vi "UFF_58.vi"(11 "array":string[](array[string])=["    58", "Transfer Function H1", "Vib & Ref1  H1 Velocity / Force", "25-Jul-01 16-14-15  ", "rubblkbrftn.svd", "NONE", "    4         3    1         0       NONE       513   2       NONE       501   2", "         5      3200         1  1.25000e+00  1.25000e+00  0.00000e+00", "        18    0    0    0            Frequency                   Hz", "        11    0    0    0             Velocity                  m/s", "        13    0    0    0                Force                    N", "         0    0    0    0                 NONE                 NONE", " -2.44772e-02 -2.29083e-02 -4.29675e-02 -3.38422e-02 -1.42753e-02 -1.87575e-02", " -4.10837e-02 -9.69093e-02 -2.05625e-01 -1.49768e-01 -3.44395e-01  1.65721e-01", " -1.09695e-01  3.16244e-01  2.64647e-01 -3.79660e-01 -3.12266e-02  6.21503e-02", " -3.37903e-02  5.86053e-02 -1.27031e-02  7.12610e-02  8.31891e-03  5.38217e-02", "  2.07081e-02  4.42556e-02  1.68963e-02  2.46244e-02  2.45377e-04 -1.47570e-02", " -5.97549e-02  3.47108e-02 -1.52918e-02  4.27029e-02 -1.50761e-02  4.24537e-02", " -5.81629e-03  3.90005e-02 -9.52282e-03  2.12302e-02 -1.48471e-02  3.79965e-02", " -6.36889e-03  4.28727e-02  1.19483e-03  3.87167e-02 -5.26405e-03  2.65269e-02", " -6.60730e-03  3.47906e-02  7.59866e-04  3.38277e-02 -1.54237e-03  3.24441e-02", "  1.03543e-03  3.03496e-02  3.38132e-03  3.12400e-02  6.82404e-03  2.80844e-02", "  6.40410e-03  2.41087e-02  4.76068e-03  2.30825e-02  4.81669e-03  2.17997e-02", "  4.57283e-03  2.07062e-02  4.58951e-03  1.95397e-02  4.21995e-03  1.79763e-02", "  3.77206e-03  1.86075e-02  3.65505e-03  1.45262e-02  8.31854e-03  1.77252e-02", "  4.44066e-04  1.54022e-02  2.11637e-03  1.37485e-02  1.98206e-03  1.44290e-02", "  8.26905e-04  1.30683e-02  8.12047e-04  1.29353e-02  9.44722e-04  1.27583e-02", "  7.80146e-04  1.20994e-02  6.20840e-04  1.14556e-02  1.53683e-04  1.13300e-02", " -1.26091e-04  1.08185e-02 -4.79234e-05  1.05322e-02 -2.48779e-04  1.01732e-02", " -2.57901e-04  9.65408e-03 -2.34030e-04  9.21830e-03 -6.76051e-04  8.78385e-03", " -4.73517e-04  8.30843e-03 -6.25769e-04  7.97665e-03 -8.67610e-04  7.67506e-03", " -8.06777e-04  7.30798e-03 -8.69391e-04  6.83099e-03 -1.08317e-03  6.43512e-03", " -1.04846e-03  6.14125e-03 -1.11451e-03  5.65235e-03 -1.40155e-03  5.38275e-03", " -1.08489e-03  5.29333e-03 -1.25805e-03  4.60217e-03 -1.34644e-03  4.25631e-03", " -1.42998e-03  3.83266e-03 -1.58892e-03  3.48706e-03 -1.49756e-03  3.32678e-03", " -1.65587e-03  2.96426e-03 -1.45823e-03  2.70408e-03 -1.36304e-03  2.35338e-03", " -1.40112e-03  2.03333e-03 -1.35197e-03  1.67269e-03 -1.33700e-03  1.33033e-03", " -1.38712e-03  1.02474e-03 -1.35330e-03  7.04625e-04 -1.34168e-03  3.02493e-04", " -1.31492e-03  4.42537e-05 -1.24354e-03 -2.61606e-04 -1.31045e-03 -5.85098e-04", " -1.23041e-03 -8.40868e-04 -1.19052e-03 -1.14186e-03 -1.15886e-03 -1.45960e-03", " -1.13493e-03 -1.81665e-03 -1.19200e-03 -2.09698e-03 -1.17228e-03 -2.32472e-03", " -1.13574e-03 -2.58351e-03 -1.05089e-03 -2.89408e-03 -1.02939e-03 -3.20176e-03", " -1.01978e-03 -3.53409e-03 -1.05770e-03 -3.85076e-03 -1.01618e-03 -4.15908e-03", " -1.05827e-03 -4.51371e-03 -1.05969e-03 -4.91698e-03 -1.11136e-03 -5.40058e-03", " -1.33444e-03 -6.24271e-03 -2.02819e-03 -7.93219e-03 -1.20950e-02 -1.05859e-02", " -1.23938e-03 -7.21660e-04 -5.88633e-04 -3.52608e-03 -6.26043e-04 -4.70434e-03", " -6.49080e-04 -5.59269e-03 -7.90585e-04 -6.39017e-03 -1.05691e-03 -7.20279e-03", " -1.49888e-03 -8.30801e-03 -2.48368e-03 -1.00025e-02 -5.73948e-03 -1.28778e-02", " -2.03627e-02 -1.04256e-02 -6.41621e-03  7.27220e-03 -1.12501e-03  1.48627e-03", " -3.76965e-04 -1.26116e-03 -1.63673e-04 -2.42729e-03 -1.05605e-04 -3.32438e-03", " -6.28148e-05 -3.94602e-03 -3.65379e-05 -4.41773e-03 -7.14368e-05 -4.92328e-03", " -1.65773e-04 -5.23990e-03 -1.11121e-04 -5.54384e-03 -8.62734e-05 -5.91084e-03", " -2.38965e-04 -6.23595e-03 -2.93454e-04 -6.49276e-03 -3.54876e-04 -6.72432e-03", " -3.84247e-04 -7.01755e-03 -4.26231e-04 -7.26887e-03 -4.68079e-04 -7.50110e-03", " -5.50005e-04 -7.74349e-03 -5.38855e-04 -8.08263e-03 -6.78949e-04 -8.27364e-03", " -8.23516e-04 -8.55511e-03 -9.11479e-04 -8.86012e-03 -1.02952e-03 -9.13512e-03", " -1.11435e-03 -9.40279e-03 -1.19906e-03 -9.71888e-03 -1.30383e-03 -1.00523e-02", " -1.36543e-03 -1.04218e-02 -1.57358e-03 -1.07785e-02 -1.75437e-03 -1.12336e-02", " -1.88485e-03 -1.17369e-02 -2.10051e-03 -1.23583e-02 -2.36793e-03 -1.30437e-02", " -2.70218e-03 -1.39592e-02 -3.36617e-03 -1.52043e-02 -4.49803e-03 -1.69481e-02", " -7.14550e-03 -1.96814e-02 -1.57230e-02 -2.20960e-02 -2.58180e-02 -4.42617e-03", " -9.63047e-03  1.52591e-03 -4.43568e-03 -2.90013e-03 -2.98325e-03 -5.90925e-03", " -2.44875e-03 -8.00737e-03 -2.13586e-03 -1.00147e-02 -1.92453e-03 -1.26817e-02", " -1.76613e-03 -2.12119e-02 -7.24883e-03  5.92566e-03 -3.74617e-03 -5.30464e-03", " -3.30943e-03 -7.83662e-03 -3.18143e-03 -9.17002e-03 -3.20382e-03 -9.99452e-03", " -3.19734e-03 -1.07628e-02 -3.28018e-03 -1.14148e-02 -3.29655e-03 -1.19787e-02", " -3.43484e-03 -1.25632e-02 -3.52232e-03 -1.31156e-02 -3.64706e-03 -1.36735e-02", " -3.81272e-03 -1.42435e-02 -3.98651e-03 -1.48962e-02 -4.28839e-03 -1.55744e-02", " -4.73988e-03 -1.63534e-02 -5.41169e-03 -1.72000e-02 -6.50653e-03 -1.81974e-02", " -8.50081e-03 -1.89605e-02 -1.19563e-02 -1.84867e-02 -1.50322e-02 -1.39329e-02", " -1.17922e-02 -8.52909e-03 -7.38661e-03 -8.54031e-03 -5.26808e-03 -1.01477e-02", " -4.33988e-03 -1.15359e-02 -3.94343e-03 -1.26208e-02 -3.68874e-03 -1.35184e-02", " -3.59556e-03 -1.42918e-02 -3.53950e-03 -1.50204e-02 -3.54120e-03 -1.56990e-02", " -3.66517e-03 -1.63109e-02 -3.76233e-03 -1.69646e-02 -4.06571e-03 -1.76060e-02", " -4.67375e-03 -1.81043e-02 -5.63994e-03 -1.81153e-02 -5.82565e-03 -1.71055e-02", " -4.78886e-03 -1.67297e-02 -4.09323e-03 -1.73630e-02 -3.77438e-03 -1.80717e-02", " -3.66661e-03 -1.86264e-02 -3.69405e-03 -1.91967e-02 -3.71520e-03 -1.97032e-02", " -3.75605e-03 -2.01873e-02 -3.80802e-03 -2.07023e-02 -3.86758e-03 -2.11635e-02", " -3.99270e-03 -2.16438e-02 -4.05359e-03 -2.21996e-02 -4.11825e-03 -2.27676e-02", " -4.29490e-03 -2.32739e-02 -4.49758e-03 -2.38733e-02 -4.62193e-03 -2.44581e-02", " -4.89301e-03 -2.50757e-02 -5.19500e-03 -2.57487e-02 -5.50594e-03 -2.64442e-02", " -5.94359e-03 -2.71775e-02 -6.34837e-03 -2.78944e-02 -6.91380e-03 -2.87559e-02", " -7.54417e-03 -2.95287e-02 -8.27267e-03 -3.04020e-02 -9.13440e-03 -3.12990e-02", " -1.00955e-02 -3.20989e-02 -1.10113e-02 -3.29445e-02 -1.17967e-02 -3.44834e-02", " -1.40662e-02 -3.64828e-02 -1.68924e-02 -3.76885e-02 -2.02288e-02 -3.84895e-02", " -2.42325e-02 -3.89596e-02 -2.90266e-02 -3.84061e-02 -3.44746e-02 -3.64698e-02", " -3.98883e-02 -3.23191e-02 -4.40884e-02 -2.57568e-02 -4.54900e-02 -1.76443e-02", " -4.36220e-02 -9.60640e-03 -3.92332e-02 -3.45144e-03 -3.38866e-02  2.53065e-04", " -2.87841e-02  1.94572e-03 -2.43773e-02  2.25328e-03 -2.10154e-02  2.17488e-03", " -1.86945e-02  2.88077e-03 -5.62906e-03  6.15677e-03 -9.93487e-03 -4.96888e-03", " -1.02003e-02 -5.51842e-03 -9.57993e-03 -6.41793e-03 -9.04119e-03 -7.43680e-03", " -8.50619e-03 -8.47237e-03 -8.10374e-03 -9.36749e-03 -8.21788e-03 -1.04090e-02", " -7.44681e-03 -1.11083e-02 -7.18344e-03 -1.19531e-02 -7.04892e-03 -1.27485e-02", " -6.89813e-03 -1.35535e-02 -6.77479e-03 -1.41792e-02 -6.71576e-03 -1.49122e-02", " -6.66610e-03 -1.56136e-02 -6.66629e-03 -1.62581e-02 -6.67076e-03 -1.69575e-02", " -6.75997e-03 -1.73613e-02 -6.74102e-03 -1.79581e-02 -6.77823e-03 -1.86114e-02", " -6.83602e-03 -1.92382e-02 -6.82591e-03 -1.97828e-02 -6.95018e-03 -2.02996e-02", " -7.03098e-03 -2.08726e-02 -7.02040e-03 -2.13344e-02 -7.00646e-03 -2.19325e-02", " -7.15722e-03 -2.24489e-02 -7.19436e-03 -2.29629e-02 -7.26307e-03 -2.35126e-02", " -7.29949e-03 -2.40669e-02 -7.35627e-03 -2.46236e-02 -7.41866e-03 -2.52008e-02", " -7.48846e-03 -2.57537e-02 -7.54766e-03 -2.62943e-02 -7.63091e-03 -2.68651e-02", " -7.75367e-03 -2.74608e-02 -7.79623e-03 -2.80148e-02 -7.88156e-03 -2.86223e-02", " -8.02096e-03 -2.92283e-02 -8.13623e-03 -2.98830e-02 -8.29750e-03 -3.04751e-02", " -8.39950e-03 -3.10903e-02 -8.60213e-03 -3.17348e-02 -8.73934e-03 -3.23658e-02", " -8.93850e-03 -3.29361e-02 -9.09092e-03 -3.34972e-02 -9.24790e-03 -3.40572e-02", " -9.45854e-03 -3.46233e-02 -9.57105e-03 -3.51911e-02 -9.69044e-03 -3.57782e-02", " -9.85754e-03 -3.63402e-02 -9.95644e-03 -3.68907e-02 -1.00737e-02 -3.75205e-02", " -1.01032e-02 -3.81506e-02 -1.01629e-02 -3.87999e-02 -1.01290e-02 -3.94921e-02", " -1.03337e-02 -4.02005e-02 -1.03863e-02 -4.09924e-02 -1.03933e-02 -4.18105e-02", " -1.04890e-02 -4.27278e-02 -1.05516e-02 -4.36220e-02 -1.06300e-02 -4.45887e-02", " -1.06859e-02 -4.56587e-02 -1.08327e-02 -4.68403e-02 -1.09898e-02 -4.81027e-02", " -1.11498e-02 -4.94590e-02 -1.13276e-02 -5.09122e-02 -1.14029e-02 -5.27525e-02", " -1.16788e-02 -5.48425e-02 -1.19936e-02 -5.75013e-02 -1.24706e-02 -6.09365e-02", " -1.31082e-02 -6.54490e-02 -1.41252e-02 -7.30632e-02 -1.72413e-02 -8.79317e-02", " -3.56330e-02 -1.33098e-01 -1.94325e-01  1.62296e-01 -2.40660e-02  3.59303e-03", " -1.70369e-02 -1.69023e-02 -1.61434e-02 -2.88090e-02 -1.58284e-02 -3.46086e-02", " -1.55154e-02 -3.88141e-02 -1.56474e-02 -4.18453e-02 -1.57677e-02 -4.42634e-02", " -1.59534e-02 -4.65386e-02 -1.61822e-02 -4.82171e-02 -1.63574e-02 -5.00098e-02", " -1.66041e-02 -5.16709e-02 -1.68711e-02 -5.32608e-02 -1.71819e-02 -5.49380e-02", " -1.76113e-02 -5.64944e-02 -1.80433e-02 -5.80203e-02 -1.85323e-02 -5.95894e-02", " -1.89794e-02 -6.11846e-02 -1.95432e-02 -6.28453e-02 -2.01533e-02 -6.45275e-02", " -2.07703e-02 -6.62862e-02 -2.15261e-02 -6.80623e-02 -2.23303e-02 -6.99359e-02", " -2.31877e-02 -7.19570e-02 -2.42232e-02 -7.40232e-02 -2.51985e-02 -7.61317e-02", " -2.62571e-02 -7.84061e-02 -2.74800e-02 -8.09735e-02 -2.89198e-02 -8.37859e-02", " -3.04736e-02 -8.67033e-02 -3.22243e-02 -9.00349e-02 -3.42317e-02 -9.36897e-02", " -3.64752e-02 -9.82037e-02 -3.95659e-02 -1.03537e-01 -4.35301e-02 -1.10161e-01", " -4.91657e-02 -1.18539e-01 -5.74648e-02 -1.29695e-01 -7.17279e-02 -1.46891e-01", " -1.04661e-01 -1.76312e-01 -2.31679e-01 -2.16735e-01 -2.59316e-01  2.41641e-01", " -2.27568e-02  4.55346e-02 -2.83313e-02 -2.48587e-02 -3.79707e-02 -4.39220e-02", " -4.14038e-02 -5.38401e-02 -4.17791e-02 -6.22446e-02 -4.21895e-02 -7.10907e-02", " -4.42248e-02 -7.99801e-02 -4.74061e-02 -8.83440e-02 -5.12458e-02 -9.60706e-02", " -5.58756e-02 -1.03902e-01 -6.13818e-02 -1.11739e-01 -6.79614e-02 -1.19732e-01", " -7.56878e-02 -1.27925e-01 -8.49835e-02 -1.36360e-01 -9.60897e-02 -1.45078e-01", " -1.09592e-01 -1.54129e-01 -1.26190e-01 -1.63099e-01 -1.46817e-01 -1.71635e-01", " -1.72724e-01 -1.78547e-01 -2.05044e-01 -1.82293e-01 -2.44733e-01 -1.79396e-01", " -2.91535e-01 -1.65133e-01 -3.41823e-01 -1.32903e-01 -3.85675e-01 -7.77070e-02", " -4.09599e-01 -1.90486e-03 -4.02517e-01  8.25842e-02 -3.61983e-01  1.59619e-01", " -2.95503e-01  2.10501e-01 -2.23672e-01  2.26437e-01 -1.65271e-01  2.16699e-01", " -1.24944e-01  1.95551e-01 -9.99964e-02  1.72551e-01 -8.58762e-02  1.53091e-01", " -7.69245e-02  1.39271e-01 -6.84614e-02  1.28972e-01 -6.03414e-02  1.19212e-01", " -5.31187e-02  1.08461e-01 -4.86226e-02  9.76905e-02 -4.68242e-02  8.74568e-02", " -4.78313e-02  7.87931e-02 -5.12034e-02  7.30068e-02 -5.55264e-02  7.14771e-02", " -5.76973e-02  7.48299e-02 -5.44775e-02  8.03326e-02 -4.61364e-02  8.31710e-02", " -3.65290e-02  8.14325e-02 -2.85759e-02  7.63912e-02 -2.27087e-02  7.00340e-02", " -1.86698e-02  6.34206e-02 -1.59849e-02  5.70071e-02 -1.41648e-02  5.09243e-02", " -1.29612e-02  4.52843e-02 -1.23344e-02  3.99549e-02 -1.19340e-02  3.50043e-02", " -1.18560e-02  3.02953e-02 -1.19671e-02  2.58074e-02 -1.22249e-02  2.15115e-02", " -1.25806e-02  1.74006e-02 -1.32436e-02  1.33647e-02 -1.38553e-02  9.34838e-03", " -1.46997e-02  5.54821e-03 -1.56013e-02  1.68279e-03 -1.66801e-02 -2.22447e-03", " -1.78547e-02 -6.09856e-03 -1.91977e-02 -9.98628e-03 -2.07270e-02 -1.39586e-02", " -2.24233e-02 -1.80041e-02 -2.42883e-02 -2.21864e-02 -2.63785e-02 -2.64944e-02", " -2.87474e-02 -3.09659e-02 -3.14932e-02 -3.57085e-02 -3.45868e-02 -4.06271e-02", " -3.82280e-02 -4.59076e-02 -4.23731e-02 -5.14185e-02 -4.72923e-02 -5.73286e-02", " -5.30239e-02 -6.36349e-02 -5.98606e-02 -7.03714e-02 -6.80793e-02 -7.74754e-02", " -7.80248e-02 -8.50566e-02 -9.02106e-02 -9.31085e-02 -1.05412e-01 -1.01248e-01", " -1.24645e-01 -1.09144e-01 -1.49159e-01 -1.15817e-01 -1.80562e-01 -1.19417e-01", " -2.20179e-01 -1.16376e-01 -2.68248e-01 -1.00886e-01 -3.20767e-01 -6.40679e-02", " -3.64451e-01  2.01733e-03 -3.76837e-01  9.29822e-02 -3.42978e-01  1.82841e-01", " -2.75844e-01  2.41738e-01 -2.03589e-01  2.62933e-01 -1.43777e-01  2.58620e-01", " -9.99062e-02  2.42536e-01 -6.89811e-02  2.22755e-01 -4.76235e-02  2.03278e-01", " -3.25788e-02  1.85480e-01 -2.18341e-02  1.69549e-01 -1.41350e-02  1.55551e-01", " -8.43137e-03  1.43241e-01 -4.14280e-03  1.32222e-01 -9.31549e-04  1.22446e-01", "  1.52311e-03  1.13596e-01  3.33610e-03  1.05596e-01  4.72895e-03  9.82302e-02", "  5.80640e-03  9.13623e-02  6.57661e-03  8.49874e-02  7.09451e-03  7.88745e-02", "  7.48204e-03  7.29451e-02  7.69199e-03  6.71450e-02  7.75508e-03  6.13431e-02", "  8.04777e-03  5.52566e-02  8.12843e-03  4.77653e-02  7.14085e-03  3.94013e-02", "  5.24321e-03  2.91639e-02  1.33287e-03  1.53849e-02 -7.58339e-03 -7.68142e-03", " -4.41354e-02  2.11962e-02 -7.32219e-02 -5.57166e-02 -2.75757e-01  7.20481e-02", " -5.68607e-02  1.76528e-01 -1.72677e-02  1.25996e-01 -9.26297e-03  1.04443e-01", " -4.60809e-03  9.39370e-02 -4.25354e-04  8.57501e-02  1.94335e-03  7.87876e-02", "  3.36414e-03  7.31486e-02  4.11329e-03  6.83924e-02  4.52444e-03  6.45397e-02", "  4.89469e-03  6.12092e-02  5.12606e-03  5.82901e-02  5.17733e-03  5.56310e-02", "  5.25150e-03  5.32135e-02  5.24259e-03  5.09776e-02  5.19958e-03  4.89898e-02", "  5.17268e-03  4.71235e-02  5.10804e-03  4.53449e-02  4.97970e-03  4.37028e-02", "  4.89549e-03  4.21339e-02  4.77411e-03  4.05814e-02  4.61617e-03  3.92065e-02", "  4.47773e-03  3.78701e-02  4.28973e-03  3.65645e-02  4.11851e-03  3.53440e-02", "  3.95208e-03  3.41527e-02  3.75195e-03  3.30220e-02  3.61893e-03  3.19111e-02", "  3.39043e-03  3.08182e-02  3.22890e-03  2.97863e-02  3.01094e-03  2.88163e-02", "  2.80494e-03  2.78735e-02  2.62512e-03  2.68830e-02  2.42577e-03  2.59799e-02", "  2.23766e-03  2.51243e-02  2.05004e-03  2.42040e-02  1.86563e-03  2.33187e-02", "  1.66073e-03  2.24668e-02  1.45658e-03  2.16522e-02  1.22753e-03  2.08519e-02", "  1.00114e-03  2.00100e-02  8.58613e-04  1.92113e-02  6.61846e-04  1.83653e-02", "  4.65438e-04  1.75309e-02  2.51143e-04  1.66827e-02  1.01465e-05  1.58675e-02", " -2.57019e-04  1.50011e-02 -5.38876e-04  1.41575e-02 -7.91532e-04  1.32718e-02", " -1.11660e-03  1.23502e-02 -1.44712e-03  1.14330e-02 -1.84932e-03  1.03891e-02", " -2.39113e-03  9.18251e-03 -3.16192e-03  7.67715e-03 -4.86657e-03  5.36725e-03", " -1.45768e-02  1.21483e-03 -3.90432e-04  1.77915e-02 -1.00483e-02  1.11625e-02", " -3.26333e-03  1.07501e-02 -3.14273e-03  8.75520e-03 -3.37219e-03  7.38487e-03", " -3.71116e-03  6.23558e-03 -4.09147e-03  5.17226e-03 -4.49609e-03  4.23650e-03", " -4.81853e-03  3.26311e-03 -5.21709e-03  2.39680e-03 -5.63970e-03  1.52901e-03", " -6.06179e-03  6.51886e-04 -6.46068e-03 -2.13497e-04 -6.89853e-03 -1.07038e-03", " -7.36264e-03 -1.97502e-03 -7.87718e-03 -2.87764e-03 -8.32877e-03 -3.75494e-03", " -8.90257e-03 -4.71284e-03 -9.42148e-03 -5.65225e-03 -9.99974e-03 -6.64615e-03", " -1.06323e-02 -7.58817e-03 -1.12696e-02 -8.56287e-03 -1.20152e-02 -9.58636e-03", " -1.27166e-02 -1.06497e-02 -1.35291e-02 -1.17437e-02 -1.43998e-02 -1.28644e-02", " -1.53590e-02 -1.40137e-02 -1.64690e-02 -1.51550e-02 -1.76461e-02 -1.63639e-02", " -1.89206e-02 -1.75686e-02 -2.03845e-02 -1.88185e-02 -2.20184e-02 -2.00305e-02", " -2.38316e-02 -2.12621e-02 -2.59244e-02 -2.24604e-02 -2.82787e-02 -2.35495e-02", " -3.09924e-02 -2.44998e-02 -3.40601e-02 -2.52507e-02 -3.75872e-02 -2.56044e-02", " -4.15365e-02 -2.54631e-02 -4.59358e-02 -2.44786e-02 -5.05366e-02 -2.23059e-02", " -5.48803e-02 -1.86219e-02 -5.83236e-02 -1.33781e-02 -5.99787e-02 -6.73715e-03", " -5.89301e-02  2.38699e-04 -5.52389e-02  6.21406e-03 -4.97927e-02  1.00381e-02", " -4.38779e-02  1.12665e-02 -3.86156e-02  1.03821e-02 -3.44773e-02  7.99521e-03", " -3.16856e-02  4.87389e-03 -3.01255e-02  1.38791e-03 -2.97564e-02 -2.11290e-03", " -3.03036e-02 -5.26933e-03 -3.18358e-02 -7.84481e-03 -3.40524e-02 -9.37536e-03", " -3.63046e-02 -9.55451e-03 -3.75135e-02 -8.47566e-03 -3.69672e-02 -7.21161e-03", " -3.51840e-02 -7.07436e-03 -3.32315e-02 -8.51651e-03 -3.18885e-02 -1.08697e-02", " -3.12577e-02 -1.38271e-02 -3.13139e-02 -1.70065e-02 -3.19315e-02 -2.02184e-02", " -3.29899e-02 -2.34024e-02 -3.44352e-02 -2.65628e-02 -3.61594e-02 -2.96841e-02", " -3.82810e-02 -3.28203e-02 -4.06682e-02 -3.59862e-02 -4.33938e-02 -3.92115e-02", " -4.65107e-02 -4.23652e-02 -5.00415e-02 -4.56365e-02 -5.40804e-02 -4.90311e-02", " -5.85747e-02 -5.23697e-02 -6.37557e-02 -5.57913e-02 -6.96608e-02 -5.92570e-02", " -7.65282e-02 -6.26068e-02 -8.43873e-02 -6.58132e-02 -9.34797e-02 -6.86842e-02", " -1.04068e-01 -7.09071e-02 -1.16237e-01 -7.23685e-02 -1.30322e-01 -7.25378e-02", " -1.46356e-01 -7.03893e-02 -1.64461e-01 -6.55453e-02 -1.84219e-01 -5.62721e-02", " -2.04804e-01 -4.18031e-02 -2.24825e-01 -1.99238e-02 -2.41407e-01  1.05910e-02", " -2.50383e-01  5.03290e-02 -2.45836e-01  9.92472e-02 -2.17380e-01  1.52610e-01", " -1.56721e-01  1.92964e-01 -6.65290e-02  1.83351e-01 -1.47605e-02  1.08646e-01", " -5.13102e-02  4.23024e-02 -5.32718e-02  1.15006e-02 -9.89055e-02 -1.11564e-02", " -1.43895e-01 -9.34384e-03 -1.84351e-01  1.27934e-02 -2.11200e-01  5.17359e-02", " -2.16291e-01  9.83653e-02 -2.01338e-01  1.40986e-01 -1.73522e-01  1.69203e-01", " -1.43039e-01  1.83377e-01 -1.16228e-01  1.86685e-01 -9.46651e-02  1.84394e-01", " -7.82604e-02  1.79931e-01 -6.57240e-02  1.75357e-01 -5.51525e-02  1.71621e-01", " -4.48700e-02  1.68580e-01 -3.46705e-02  1.64855e-01 -2.46676e-02  1.60008e-01", " -1.57069e-02  1.53769e-01 -8.41623e-03  1.46636e-01 -2.81037e-03  1.39282e-01", "  1.43142e-03  1.32189e-01  4.63703e-03  1.25530e-01  6.89588e-03  1.19328e-01", "  8.52459e-03  1.13772e-01  9.78263e-03  1.08640e-01  1.05958e-02  1.03988e-01", "  1.12568e-02  9.96551e-02  1.16432e-02  9.56900e-02  1.19348e-02  9.20537e-02", "  1.21344e-02  8.87438e-02  1.21816e-02  8.55622e-02  1.20985e-02  8.26659e-02", "  1.20358e-02  7.98995e-02  1.18263e-02  7.73074e-02  1.15845e-02  7.48828e-02", "  1.12805e-02  7.25941e-02  1.08617e-02  7.04233e-02  1.04252e-02  6.83774e-02", "  9.84184e-03  6.64683e-02  9.23935e-03  6.47672e-02  8.48506e-03  6.32090e-02", "  7.68083e-03  6.18489e-02  6.92759e-03  6.08219e-02  6.21752e-03  6.00960e-02", "  5.70667e-03  5.96455e-02  5.54668e-03  5.93558e-02  5.76831e-03  5.90431e-02", "  6.29679e-03  5.85396e-02  6.89330e-03  5.76785e-02  7.48417e-03  5.66367e-02", "  7.90988e-03  5.54089e-02  8.20194e-03  5.41257e-02  8.36320e-03  5.27693e-02", "  8.44770e-03  5.14125e-02  8.41802e-03  5.01470e-02  8.30937e-03  4.88651e-02", "  8.10841e-03  4.76374e-02  7.88699e-03  4.64506e-02  7.61947e-03  4.53183e-02", "  7.38338e-03  4.41636e-02  7.03748e-03  4.30694e-02  6.63279e-03  4.19657e-02", "  6.25468e-03  4.09080e-02  5.79028e-03  3.98809e-02  5.29288e-03  3.88174e-02", "  4.70311e-03  3.77722e-02  4.03381e-03  3.67404e-02  3.30579e-03  3.57517e-02", "  2.44903e-03  3.47418e-02  1.49192e-03  3.37926e-02  3.16852e-04  3.28983e-02", " -1.05155e-03  3.21223e-02 -2.73285e-03  3.15499e-02 -4.85751e-03  3.13326e-02", " -7.44774e-03  3.18311e-02 -1.06179e-02  3.44799e-02 -1.06187e-02  4.20971e-02", "  3.00040e-03  4.47454e-02  6.76422e-03  2.97673e-02 -6.43578e-04  1.99213e-02", " -1.67899e-02  7.55626e-03 -2.32186e-02  7.04904e-02 -7.44162e-03  4.34349e-02", " -9.51240e-03  3.97603e-02 -1.08674e-02  4.01615e-02 -1.08953e-02  4.16893e-02", " -9.87852e-03  4.29225e-02 -8.32210e-03  4.34996e-02 -6.87281e-03  4.32430e-02", " -5.91587e-03  4.25369e-02 -5.50414e-03  4.16274e-02 -5.58586e-03  4.07991e-02", " -6.14856e-03  4.01878e-02 -6.96923e-03  4.00957e-02 -7.99888e-03  4.05651e-02", " -8.72679e-03  4.15840e-02 -8.99120e-03  4.32807e-02 -8.50700e-03  4.50880e-02", " -7.18309e-03  4.68170e-02 -5.25878e-03  4.79235e-02 -3.07582e-03  4.83558e-02", " -9.95834e-04  4.81150e-02  8.75158e-04  4.74167e-02  2.36073e-03  4.64030e-02", "  3.55639e-03  4.52390e-02  4.42304e-03  4.40239e-02  5.09416e-03  4.28431e-02", "  5.58488e-03  4.16205e-02  5.89232e-03  4.05016e-02  6.09706e-03  3.94142e-02", "  6.19783e-03  3.83782e-02  6.17611e-03  3.74410e-02  6.11632e-03  3.65143e-02", "  5.91904e-03  3.56542e-02  5.78905e-03  3.48646e-02  5.49505e-03  3.40989e-02", "  5.21990e-03  3.34057e-02  4.90616e-03  3.27469e-02  4.53064e-03  3.21491e-02", "  4.09742e-03  3.15990e-02  3.66159e-03  3.09963e-02  3.16905e-03  3.05693e-02", "  2.62064e-03  3.01505e-02  2.04847e-03  2.97764e-02  1.44979e-03  2.94967e-02", "  7.25556e-04  2.93647e-02  1.62217e-05  2.92545e-02 -6.97813e-04  2.93078e-02", " -1.45818e-03  2.94997e-02 -2.15472e-03  2.98434e-02 -2.85110e-03  3.03675e-02", " -3.45972e-03  3.10743e-02 -3.89954e-03  3.20479e-02 -4.10696e-03  3.32043e-02", " -3.96485e-03  3.44875e-02 -3.47380e-03  3.57993e-02 -2.48352e-03  3.70118e-02", " -1.15689e-03  3.79910e-02  4.33576e-04  3.85377e-02  2.18644e-03  3.86245e-02", "  3.87628e-03  3.82296e-02  5.37911e-03  3.75890e-02  6.62386e-03  3.65802e-02", "  7.62765e-03  3.54739e-02  8.40772e-03  3.42890e-02  8.93006e-03  3.30627e-02", "  9.32949e-03  3.18093e-02  9.59017e-03  3.05849e-02  9.70092e-03  2.93460e-02", "  9.64260e-03  2.81625e-02  9.56740e-03  2.68987e-02  9.32409e-03  2.55425e-02", "  8.83511e-03  2.39712e-02  7.96230e-03  2.22240e-02  6.52250e-03  2.04837e-02", "  4.44411e-03  1.51225e-02 -7.51501e-03  1.99506e-02 -5.88622e-03  3.34510e-02", "  3.09228e-03  3.41454e-02  6.21906e-03  3.14336e-02  7.39884e-03  2.93985e-02", "  7.97300e-03  2.79033e-02  8.12127e-03  2.66218e-02  8.09940e-03  2.56057e-02", "  8.02761e-03  2.48271e-02  7.91039e-03  2.40731e-02  7.78201e-03  2.34743e-02", "  7.65646e-03  2.28755e-02  7.56805e-03  2.23087e-02  7.44959e-03  2.17816e-02", "  7.29364e-03  2.13158e-02  7.14524e-03  2.08284e-02  7.03786e-03  2.03555e-02", "  6.85115e-03  1.99036e-02  6.65956e-03  1.94526e-02  6.46119e-03  1.90453e-02", "  6.26342e-03  1.86128e-02  6.07117e-03  1.82303e-02  5.81833e-03  1.78214e-02", "  5.58592e-03  1.74393e-02  5.37784e-03  1.71297e-02  5.17702e-03  1.67577e-02", "  4.93984e-03  1.63727e-02  4.70603e-03  1.60488e-02  4.51636e-03  1.57717e-02", "  4.27555e-03  1.53871e-02  4.03940e-03  1.50554e-02  3.79389e-03  1.47416e-02", "  3.49398e-03  1.43875e-02  3.23353e-03  1.40725e-02  3.00218e-03  1.37729e-02", "  2.73499e-03  1.34835e-02  2.46769e-03  1.31592e-02  2.15677e-03  1.28625e-02", "  1.90676e-03  1.25682e-02  1.60560e-03  1.22556e-02  1.29719e-03  1.19682e-02", "  1.02583e-03  1.16246e-02  6.65817e-04  1.13146e-02  3.42913e-04  1.09096e-02", " -2.83669e-05  1.05785e-02 -3.79577e-04  1.02025e-02 -8.00840e-04  9.82547e-03", " -1.25904e-03  9.43080e-03 -1.71018e-03  9.03168e-03 -2.22057e-03  8.65338e-03", " -2.83926e-03  8.27967e-03 -3.48037e-03  7.89241e-03 -4.12397e-03  7.49828e-03", " -4.90570e-03  7.14847e-03 -5.70228e-03  6.81308e-03 -6.54896e-03  6.44811e-03", " -7.51660e-03  6.15994e-03 -8.59352e-03  5.88061e-03 -9.81842e-03  5.65735e-03", " -1.11486e-02  5.47747e-03 -1.26343e-02  5.41786e-03 -1.43234e-02  5.57281e-03", " -1.61618e-02  5.94904e-03 -1.81562e-02  6.64130e-03 -2.02838e-02  7.70806e-03", " -2.24639e-02  9.25824e-03 -2.45533e-02  1.15016e-02 -2.62346e-02  1.43878e-02", " -2.72586e-02  1.79205e-02 -2.73778e-02  2.19213e-02 -2.63361e-02  2.60456e-02", " -2.41019e-02  2.96448e-02 -2.09218e-02  3.24048e-02 -1.73879e-02  3.40388e-02", " -1.38445e-02  3.46269e-02 -1.06074e-02  3.43224e-02 -7.92675e-03  3.34271e-02", " -5.69629e-03  3.21594e-02 -3.97813e-03  3.07659e-02 -2.75082e-03  2.92792e-02", " -1.86793e-03  2.78230e-02 -1.26525e-03  2.64492e-02 -8.23575e-04  2.51560e-02", " -6.04430e-04  2.39951e-02 -5.70911e-04  2.28452e-02 -5.72773e-04  2.18492e-02", " -7.22486e-04  2.09514e-02 -8.54037e-04  2.01251e-02 -1.17184e-03  1.93833e-02", " -1.47543e-03  1.86940e-02 -1.82026e-03  1.81009e-02 -2.20990e-03  1.75656e-02", " -2.59962e-03  1.71339e-02 -3.13117e-03  1.68076e-02 -3.57586e-03  1.65043e-02", " -4.09479e-03  1.63273e-02 -4.56651e-03  1.62618e-02 -5.00901e-03  1.62453e-02", " -5.35585e-03  1.63818e-02 -5.68065e-03  1.65928e-02 -5.80818e-03  1.68602e-02", " -5.81355e-03  1.70771e-02 -5.77195e-03  1.72836e-02 -5.56844e-03  1.73413e-02", " -5.32495e-03  1.73658e-02 -5.03881e-03  1.71187e-02 -4.81411e-03  1.68317e-02", " -4.80766e-03  1.63730e-02 -4.90105e-03  1.59316e-02 -5.13260e-03  1.54819e-02", " -5.48317e-03  1.51879e-02 -5.97923e-03  1.49689e-02 -6.44054e-03  1.49497e-02", " -6.94811e-03  1.50677e-02 -7.27069e-03  1.53180e-02 -7.42471e-03  1.57135e-02", " -7.35685e-03  1.60616e-02 -7.12520e-03  1.63640e-02 -6.80822e-03  1.64901e-02", " -6.43583e-03  1.63805e-02 -6.08241e-03  1.61301e-02 -5.84208e-03  1.57476e-02", " -5.68913e-03  1.52396e-02 -5.62212e-03  1.47152e-02 -5.82236e-03  1.41052e-02", " -5.95526e-03  1.35929e-02 -6.29923e-03  1.30547e-02 -6.71183e-03  1.24638e-02", " -7.24961e-03  1.20094e-02 -7.77430e-03  1.16062e-02 -8.40385e-03  1.11588e-02", " -9.20234e-03  1.07709e-02 -1.00136e-02  1.04244e-02 -1.09992e-02  1.01962e-02", " -1.20415e-02  1.00235e-02 -1.31711e-02  9.96903e-03 -1.44177e-02  1.01255e-02", " -1.58237e-02  1.03938e-02 -1.72391e-02  1.09365e-02 -1.87006e-02  1.16579e-02", " -2.01364e-02  1.27412e-02 -2.15649e-02  1.40642e-02 -2.27915e-02  1.58660e-02", " -2.38125e-02  1.79136e-02 -2.45012e-02  2.03469e-02 -2.47540e-02  2.30017e-02", " -2.43849e-02  2.58424e-02 -2.34281e-02  2.87185e-02 -2.18764e-02  3.14071e-02", " -1.97052e-02  3.38953e-02 -1.68995e-02  3.59308e-02 -1.36751e-02  3.76130e-02", " -9.30834e-03  3.88497e-02 -2.79255e-03  3.90061e-02  7.43433e-03  2.97921e-02", " -5.73775e-03  1.83585e-02 -7.75351e-03  2.92047e-02 -4.44532e-03  2.14605e-02", " -1.02032e-02  2.90244e-02 -6.92222e-03  2.94759e-02 -5.71389e-03  2.94377e-02", " -4.58767e-03  2.94781e-02 -3.65680e-03  2.96045e-02 -2.39887e-03  2.97756e-02", " -8.25303e-04  3.00238e-02  1.39976e-03  3.00219e-02  4.42867e-03  2.90786e-02", "  7.82082e-03  2.63937e-02  1.01556e-02  2.10876e-02  8.53570e-03  1.42266e-02", "  2.59167e-03  9.93943e-03 -3.63903e-03  1.05305e-02 -7.15239e-03  1.35517e-02", " -8.49626e-03  1.67032e-02 -8.52841e-03  1.93834e-02 -7.74604e-03  2.13740e-02", " -6.48528e-03  2.27882e-02 -5.10074e-03  2.35451e-02 -3.71743e-03  2.37668e-02", " -2.47935e-03  2.36102e-02 -1.42497e-03  2.32678e-02 -5.76839e-04  2.26858e-02", "  5.52566e-05  2.20242e-02  6.28204e-04  2.13501e-02  9.60243e-04  2.06601e-02", "  1.20904e-03  1.99318e-02  1.39694e-03  1.92244e-02  1.45404e-03  1.85604e-02", "  1.52527e-03  1.79311e-02  1.41276e-03  1.73183e-02  1.32861e-03  1.66981e-02", "  1.14371e-03  1.62007e-02  9.68750e-04  1.56548e-02  7.42549e-04  1.51905e-02", "  4.69247e-04  1.48011e-02  2.28849e-04  1.44174e-02 -1.53633e-04  1.40639e-02", " -4.63871e-04  1.37901e-02 -7.77812e-04  1.35338e-02 -1.13930e-03  1.33193e-02", " -1.42324e-03  1.31697e-02 -1.81758e-03  1.30452e-02 -2.13845e-03  1.29420e-02", " -2.52933e-03  1.28912e-02 -2.76632e-03  1.29282e-02 -3.07552e-03  1.30208e-02", " -3.37524e-03  1.31265e-02 -3.61110e-03  1.32381e-02 -3.86262e-03  1.34390e-02", " -4.04094e-03  1.36523e-02 -4.17067e-03  1.39082e-02 -4.25210e-03  1.41194e-02", " -4.25773e-03  1.45094e-02 -4.17873e-03  1.48543e-02 -4.04927e-03  1.52288e-02", " -3.80309e-03  1.55490e-02 -3.43573e-03  1.59244e-02 -2.95065e-03  1.61137e-02", " -2.33112e-03  1.62713e-02 -1.77170e-03  1.62105e-02 -1.17033e-03  1.60699e-02", " -6.19596e-04  1.58204e-02 -1.44270e-04  1.54288e-02  2.93751e-04  1.49877e-02", "  6.25891e-04  1.45457e-02  8.85279e-04  1.40563e-02  1.06073e-03  1.35618e-02", "  1.24398e-03  1.29821e-02  1.32472e-03  1.25401e-02  1.33757e-03  1.20770e-02", "  1.39883e-03  1.15942e-02  1.38335e-03  1.11574e-02  1.37202e-03  1.06712e-02", "  1.30868e-03  1.02890e-02  1.28813e-03  9.87252e-03  1.19365e-03  9.47283e-03", "  1.04421e-03  9.02547e-03  9.36054e-04  8.65044e-03  8.51654e-04  8.29339e-03", "  6.76622e-04  7.91132e-03  5.62757e-04  7.52639e-03  3.64582e-04  7.14249e-03", "  2.29236e-04  6.77989e-03  1.31981e-05  6.44852e-03 -1.51365e-04  6.08383e-03", " -3.34855e-04  5.68262e-03 -5.69019e-04  5.42743e-03 -7.88143e-04  4.98250e-03", " -1.04429e-03  4.68449e-03 -1.22401e-03  4.41144e-03 -1.51237e-03  4.05060e-03", " -1.77913e-03  3.75307e-03 -2.05860e-03  3.43081e-03 -2.35813e-03  3.16428e-03", " -2.63999e-03  2.90791e-03 -2.90717e-03  2.52927e-03 -3.26071e-03  2.21483e-03", " -3.65567e-03  1.97705e-03 -3.97969e-03  1.63373e-03 -4.36193e-03  1.34087e-03", " -4.86722e-03  9.79818e-04 -5.35264e-03  7.07644e-04 -6.00464e-03  4.28848e-04", " -6.71622e-03  2.51217e-04 -7.57024e-03  6.13954e-05 -8.86520e-03  1.25958e-05", " -1.08394e-02  5.89838e-04 -1.35112e-02  4.05930e-03 -7.73662e-03  1.09866e-02", " -2.77687e-03  5.13862e-03 -4.00592e-03  2.18208e-03 -4.68294e-03  9.07447e-04", " -6.42302e-03  3.40186e-04 -7.00686e-03  2.38233e-03 -5.41304e-03  1.67299e-04", " -6.54011e-03 -6.56738e-04 -7.14494e-03 -9.19840e-04 -7.59506e-03 -1.11600e-03", " -8.11434e-03 -1.29479e-03 -8.52322e-03 -1.45113e-03 -8.91983e-03 -1.56141e-03", " -9.17836e-03 -1.72148e-03 -9.48642e-03 -1.80624e-03 -9.76295e-03 -1.99797e-03", " -1.00175e-02 -2.19019e-03 -1.03215e-02 -2.26146e-03 -1.05767e-02 -2.44742e-03", " -1.08396e-02 -2.56037e-03 -1.10149e-02 -2.73536e-03 -1.12444e-02 -2.92647e-03", " -1.13884e-02 -3.22299e-03 -1.16321e-02 -3.47835e-03 -1.18117e-02 -3.78368e-03", " -1.20460e-02 -4.15323e-03 -1.23330e-02 -4.56119e-03 -1.26454e-02 -4.96541e-03", " -1.30533e-02 -5.32963e-03 -1.34433e-02 -5.79288e-03 -1.38818e-02 -6.23773e-03", " -1.44533e-02 -6.71147e-03 -1.51106e-02 -7.26183e-03 -1.58302e-02 -7.70308e-03", " -1.66729e-02 -8.15451e-03 -1.76557e-02 -8.62778e-03 -1.88384e-02 -9.08889e-03", " -2.04752e-02 -9.82695e-03 -2.31649e-02 -1.02275e-02 -2.77982e-02 -9.92460e-03", " -3.74701e-02 -3.91965e-03 -1.99129e-02  2.81116e-02 -9.09408e-03  7.09068e-04", " -1.14643e-02 -2.95626e-04 -1.24053e-02 -6.08190e-03 -1.45715e-02 -7.83959e-03", " -1.60148e-02 -8.62756e-03 -1.69848e-02 -9.45676e-03 -1.80397e-02 -1.00711e-02", " -1.89506e-02 -1.06561e-02 -1.98459e-02 -1.12609e-02 -2.07405e-02 -1.18487e-02", " -2.16277e-02 -1.22567e-02 -2.25312e-02 -1.26940e-02 -2.33938e-02 -1.32365e-02", " -2.43353e-02 -1.36745e-02 -2.52691e-02 -1.41125e-02 -2.62779e-02 -1.45829e-02", " -2.72296e-02 -1.49698e-02 -2.82645e-02 -1.54095e-02 -2.94021e-02 -1.58705e-02", " -3.05031e-02 -1.63208e-02 -3.17316e-02 -1.67398e-02 -3.29550e-02 -1.71179e-02", " -3.42856e-02 -1.74994e-02 -3.56311e-02 -1.79607e-02 -3.70650e-02 -1.82881e-02", " -3.85704e-02 -1.86719e-02 -4.01321e-02 -1.89512e-02 -4.18349e-02 -1.92883e-02", " -4.35688e-02 -1.95470e-02 -4.54777e-02 -1.97903e-02 -4.73503e-02 -1.99778e-02", " -4.94689e-02 -2.01380e-02 -5.17223e-02 -2.02413e-02 -5.40508e-02 -2.02385e-02", " -5.65505e-02 -2.02177e-02 -5.91759e-02 -2.00502e-02 -6.19765e-02 -1.97162e-02", " -6.49473e-02 -1.93340e-02 -6.79811e-02 -1.87455e-02 -7.13310e-02 -1.79539e-02", " -7.47954e-02 -1.69889e-02 -7.85212e-02 -1.57028e-02 -8.23892e-02 -1.40824e-02", " -8.65285e-02 -1.21794e-02 -9.08358e-02 -9.75107e-03 -9.52889e-02 -6.80062e-03", " -9.98383e-02 -3.22144e-03 -1.04413e-01  1.02800e-03 -1.09016e-01  6.13765e-03", " -1.13273e-01  1.21498e-02 -1.17236e-01  1.90841e-02 -1.20585e-01  2.70379e-02", " -1.23003e-01  3.60291e-02 -1.24164e-01  4.58049e-02 -1.23836e-01  5.62992e-02", " -1.21815e-01  6.70976e-02 -1.17857e-01  7.77333e-02 -1.11994e-01  8.77485e-02", " -1.04467e-01  9.66312e-02 -9.54807e-02  1.03998e-01 -8.56977e-02  1.09546e-01", " -7.54604e-02  1.13295e-01 -6.53573e-02  1.15055e-01 -5.56741e-02  1.15315e-01", " -4.67829e-02  1.14223e-01 -3.87243e-02  1.12185e-01 -3.16966e-02  1.09267e-01", " -2.56222e-02  1.06051e-01 -2.04172e-02  1.02495e-01 -1.60651e-02  9.87579e-02", " -1.24334e-02  9.51725e-02 -9.47077e-03  9.17023e-02 -6.94151e-03  8.85860e-02", " -4.77150e-03  8.57714e-02 -2.78425e-03  8.34443e-02 -4.10910e-04  8.17001e-02", "  2.93701e-03  8.04770e-02  8.75024e-03  7.83007e-02  1.63349e-02  7.11256e-02", "  1.76878e-02  5.77369e-02  1.13553e-02  4.79382e-02  2.60288e-03  4.15783e-02", " -1.24178e-02  4.70220e-02 -6.76195e-03  5.37071e-02 -6.08658e-03  5.23314e-02", " -7.05642e-03  5.16767e-02 -8.39166e-03  5.17119e-02 -9.67704e-03  5.23913e-02", " -1.06575e-02  5.36575e-02 -1.13730e-02  5.53326e-02 -1.13527e-02  5.74153e-02", " -1.05922e-02  5.97640e-02 -9.01565e-03  6.20276e-02 -6.63731e-03  6.38975e-02", " -3.67309e-03  6.52532e-02 -2.68428e-04  6.58355e-02  3.20097e-03  6.56267e-02", "  6.54506e-03  6.46928e-02  9.56147e-03  6.31540e-02  1.21739e-02  6.12252e-02", "  1.43391e-02  5.90095e-02  1.61038e-02  5.66702e-02  1.75070e-02  5.42683e-02", "  1.85732e-02  5.19263e-02  1.93394e-02  4.96463e-02  1.99137e-02  4.73820e-02", "  2.02968e-02  4.53083e-02  2.05277e-02  4.33255e-02  2.06581e-02  4.13674e-02", "  2.06768e-02  3.95743e-02  2.06387e-02  3.78613e-02  2.05250e-02  3.61916e-02", "  2.03328e-02  3.46524e-02  2.01204e-02  3.31039e-02  1.98486e-02  3.16578e-02", "  1.95680e-02  3.02717e-02  1.92338e-02  2.88863e-02  1.89746e-02  2.76195e-02", "  1.85155e-02  2.63683e-02  1.81569e-02  2.50825e-02  1.77760e-02  2.38820e-02", "  1.72872e-02  2.26764e-02  1.67796e-02  2.15545e-02  1.62143e-02  2.03757e-02", "  1.56613e-02  1.93513e-02  1.50256e-02  1.83207e-02  1.44158e-02  1.72653e-02", "  1.37149e-02  1.63129e-02  1.29407e-02  1.54193e-02  1.22256e-02  1.45750e-02", "  1.13553e-02  1.37654e-02  1.05642e-02  1.30680e-02  9.82936e-03  1.23868e-02", "  9.04025e-03  1.18142e-02  8.21353e-03  1.12040e-02  7.40769e-03  1.06156e-02", "  6.64621e-03  1.00734e-02  5.80136e-03  9.61829e-03  5.01161e-03  9.17458e-03", "  4.19088e-03  8.89972e-03  3.37948e-03  8.59305e-03  2.59246e-03  8.37832e-03", "  1.82915e-03  8.21372e-03  1.14897e-03  8.16736e-03  4.86501e-04  8.10648e-03", " -6.50665e-05  8.12535e-03 -4.93288e-04  8.08960e-03 -1.03570e-03  7.97033e-03", " -1.38769e-03  7.84868e-03 -1.80209e-03  7.65546e-03 -2.33525e-03  7.50241e-03", " -2.97416e-03  7.38038e-03 -3.67107e-03  7.55457e-03 -4.17496e-03  8.04784e-03", " -4.44959e-03  8.92316e-03 -3.45062e-03  1.05517e-02  8.87138e-04  1.02943e-02", "  1.06664e-03  4.05002e-03 -2.61526e-03  3.02134e-03 -3.77736e-03  3.32864e-03", " -4.58175e-03  3.20558e-03 -5.31445e-03  3.07665e-03 -5.95714e-03  2.85111e-03", " -6.42985e-03  2.63301e-03 -6.94467e-03  2.32881e-03 -7.37671e-03  2.06442e-03", " -7.90516e-03  1.79154e-03 -8.39901e-03  1.40504e-03 -8.87225e-03  1.10287e-03", " -9.37694e-03  7.48100e-04 -9.87252e-03  3.72304e-04 -1.04287e-02 -2.88377e-05", " -1.09507e-02 -4.04016e-04 -1.15232e-02 -8.73211e-04 -1.20878e-02 -1.22077e-03", " -1.26648e-02 -1.67772e-03 -1.33139e-02 -2.06613e-03 -1.39565e-02 -2.47353e-03", " -1.45804e-02 -2.91215e-03 -1.53079e-02 -3.32568e-03 -1.60425e-02 -3.83335e-03", " -1.68022e-02 -4.30129e-03 -1.75545e-02 -4.70881e-03 -1.84051e-02 -5.20237e-03", " -1.91691e-02 -5.61442e-03 -2.00528e-02 -6.09227e-03 -2.09433e-02 -6.61411e-03", " -2.19418e-02 -7.01949e-03 -2.28924e-02 -7.49493e-03 -2.39889e-02 -7.95686e-03", " -2.50118e-02 -8.41415e-03 -2.61552e-02 -8.91684e-03 -2.73903e-02 -9.29457e-03", " -2.85954e-02 -9.86138e-03 -2.99013e-02 -1.02563e-02 -3.12179e-02 -1.06027e-02", " -3.26164e-02 -1.11375e-02 -3.41174e-02 -1.14932e-02 -3.57016e-02 -1.18643e-02", " -3.72253e-02 -1.22903e-02 -3.89684e-02 -1.27046e-02 -4.08125e-02 -1.30801e-02", " -4.27901e-02 -1.33838e-02 -4.48578e-02 -1.36732e-02 -4.70269e-02 -1.39260e-02", " -4.93606e-02 -1.41369e-02 -5.18295e-02 -1.43498e-02 -5.45557e-02 -1.43369e-02", " -5.73213e-02 -1.42224e-02 -6.03390e-02 -1.41368e-02 -6.36095e-02 -1.37765e-02", " -6.69813e-02 -1.33463e-02 -7.06731e-02 -1.26250e-02 -7.45531e-02 -1.16757e-02", " -7.86527e-02 -1.04334e-02 -8.30852e-02 -8.71431e-03 -8.76786e-02 -6.62624e-03", " -9.25533e-02 -3.97747e-03 -9.74845e-02 -7.00301e-04 -1.02587e-01  3.27323e-03", " -1.07644e-01  8.21989e-03 -1.12640e-01  1.39037e-02 -1.17189e-01  2.08035e-02", " -1.21322e-01  2.86912e-02 -1.24401e-01  3.76826e-02 -1.26395e-01  4.76286e-02", " -1.26930e-01  5.82418e-02 -1.25769e-01  6.93724e-02 -1.22662e-01  8.04725e-02", " -1.17590e-01  9.10558e-02 -1.10814e-01  1.00657e-01 -1.02658e-01  1.08846e-01", " -9.34937e-02  1.15352e-01 -8.38929e-02  1.20147e-01 -7.41728e-02  1.23193e-01", " -6.47209e-02  1.24790e-01 -5.58355e-02  1.25291e-01 -4.75488e-02  1.24607e-01", " -3.99590e-02  1.23366e-01 -3.29419e-02  1.21351e-01 -2.65554e-02  1.18999e-01", " -2.08155e-02  1.16252e-01 -1.56169e-02  1.13156e-01 -1.09139e-02  1.09664e-01", " -6.80048e-03  1.06106e-01 -3.32337e-03  1.02381e-01 -4.40237e-04  9.85148e-02", "  1.92818e-03  9.47511e-02  3.76700e-03  9.11254e-02  5.25455e-03  8.75756e-02", "  6.32176e-03  8.43179e-02  7.00779e-03  8.11874e-02  7.50694e-03  7.83110e-02", "  7.78644e-03  7.57032e-02  7.83084e-03  7.32766e-02  7.79456e-03  7.10357e-02", "  7.63180e-03  6.90636e-02  7.28780e-03  6.73006e-02  6.93120e-03  6.58471e-02", "  6.61579e-03  6.45022e-02  6.21603e-03  6.35284e-02  5.87175e-03  6.27052e-02", "  5.61792e-03  6.21222e-02  5.53392e-03  6.17878e-02  5.66842e-03  6.15331e-02", "  6.19418e-03  6.14482e-02  6.90589e-03  6.13540e-02  8.06493e-03  6.11525e-02", "  9.58522e-03  6.07446e-02  1.13046e-02  5.99262e-02  1.31578e-02  5.86053e-02", "  1.50664e-02  5.66704e-02  1.65879e-02  5.42333e-02  1.76804e-02  5.13579e-02", "  1.82297e-02  4.80988e-02  1.80228e-02  4.48487e-02  1.72499e-02  4.17855e-02", "  1.59397e-02  3.89474e-02  1.43172e-02  3.65719e-02  1.23409e-02  3.46606e-02", "  1.03555e-02  3.32709e-02  8.57287e-03  3.22645e-02  6.89411e-03  3.13160e-02", "  5.33961e-03  3.05652e-02  3.79276e-03  2.99732e-02  2.20858e-03  2.93036e-02", "  6.30916e-04  2.87917e-02 -9.12388e-04  2.83935e-02 -2.60557e-03  2.80458e-02", " -4.19967e-03  2.78117e-02 -5.96738e-03  2.77391e-02 -7.71614e-03  2.77747e-02", " -9.63616e-03  2.80858e-02 -1.16068e-02  2.85799e-02 -1.35277e-02  2.93112e-02", " -1.55048e-02  3.03612e-02 -1.74289e-02  3.18174e-02 -1.92139e-02  3.36959e-02", " -2.07978e-02  3.58736e-02 -2.21263e-02  3.86186e-02 -2.30622e-02  4.16991e-02", " -2.34965e-02  4.53718e-02 -2.31242e-02  4.95438e-02 -2.16643e-02  5.40453e-02", " -1.88459e-02  5.89417e-02 -1.40018e-02  6.36380e-02 -6.59318e-03  6.70388e-02", "  3.04408e-03  6.76874e-02  1.35724e-02  6.35305e-02  2.13645e-02  5.42785e-02", "  2.34837e-02  4.28796e-02  2.08223e-02  3.29682e-02  1.55902e-02  2.64772e-02", "  1.04652e-02  2.27118e-02  6.20703e-03  1.99209e-02  4.98324e-04  1.96474e-02", " -2.60984e-04  1.80813e-02 -4.88549e-03  1.50591e-02 -1.11212e-02  1.37279e-02", " -1.64622e-02  1.47751e-02 -2.11316e-02  1.65151e-02 -2.53855e-02  1.86753e-02", " -2.91701e-02  2.13334e-02 -3.25913e-02  2.45798e-02 -3.54188e-02  2.83422e-02", " -3.76022e-02  3.25683e-02 -3.90007e-02  3.70242e-02 -3.96775e-02  4.15917e-02", " -3.96059e-02  4.59868e-02 -3.89440e-02  5.02614e-02 -3.77176e-02  5.42056e-02", " -3.60446e-02  5.79252e-02 -3.39682e-02  6.12499e-02 -3.15291e-02  6.42449e-02", " -2.87851e-02  6.68720e-02 -2.57893e-02  6.90885e-02 -2.25950e-02  7.08514e-02", " -1.92597e-02  7.21741e-02 -1.57424e-02  7.30738e-02 -1.22158e-02  7.33055e-02", " -8.79068e-03  7.31568e-02 -5.68729e-03  7.24740e-02 -2.63665e-03  7.13009e-02", " -1.37868e-04  6.98972e-02  2.03012e-03  6.82200e-02  3.82442e-03  6.64357e-02", "  5.29122e-03  6.45392e-02  6.38384e-03  6.26310e-02  7.21195e-03  6.07581e-02", "  7.66762e-03  5.90436e-02  8.02097e-03  5.75129e-02  8.23983e-03  5.60516e-02", "  8.23763e-03  5.46599e-02  8.26331e-03  5.34671e-02  8.09672e-03  5.23141e-02", "  8.04109e-03  5.12852e-02  7.91171e-03  5.03295e-02  7.66543e-03  4.94560e-02", "  7.41706e-03  4.85772e-02  7.16275e-03  4.78065e-02  6.91682e-03  4.70148e-02", "  6.57147e-03  4.62741e-02  6.24175e-03  4.55382e-02  5.85256e-03  4.48280e-02", "  5.37911e-03  4.41772e-02  4.85922e-03  4.34927e-02  4.34859e-03  4.29241e-02", "  3.66016e-03  4.24621e-02  2.97193e-03  4.19338e-02  2.17813e-03  4.15579e-02", "  1.34991e-03  4.12414e-02  4.78995e-04  4.10249e-02 -3.73292e-04  4.09923e-02", " -1.41076e-03  4.09167e-02 -2.32870e-03  4.11042e-02 -3.30125e-03  4.13952e-02", " -4.15379e-03  4.18264e-02 -5.07029e-03  4.24070e-02 -5.90130e-03  4.31002e-02", " -6.65506e-03  4.39560e-02 -7.30347e-03  4.48290e-02 -7.74731e-03  4.59574e-02", " -8.01831e-03  4.71360e-02 -8.28175e-03  4.82447e-02 -8.26671e-03  4.95244e-02", " -8.17345e-03  5.06710e-02 -7.99611e-03  5.18230e-02 -7.58324e-03  5.30279e-02", " -7.24894e-03  5.41089e-02 -6.66914e-03  5.52400e-02 -5.96827e-03  5.63470e-02", " -5.31295e-03  5.73947e-02 -4.31585e-03  5.84780e-02 -3.26525e-03  5.95219e-02", " -2.09035e-03  6.05119e-02 -7.19926e-04  6.13448e-02  7.54299e-04  6.20477e-02", "  2.54680e-03  6.26333e-02  4.39091e-03  6.29116e-02  6.28194e-03  6.29077e-02", "  8.10515e-03  6.26583e-02  9.95929e-03  6.20923e-02  1.16130e-02  6.13182e-02", "  1.31685e-02  6.03935e-02  1.45369e-02  5.91928e-02  1.56856e-02  5.79878e-02", "  1.65736e-02  5.66485e-02  1.73321e-02  5.52683e-02  1.80255e-02  5.38891e-02", "  1.84311e-02  5.25611e-02  1.85948e-02  5.12510e-02  1.87983e-02  4.99859e-02", "  1.88284e-02  4.86440e-02  1.87343e-02  4.75119e-02  1.85617e-02  4.63877e-02", "  1.82940e-02  4.53518e-02  1.79986e-02  4.42743e-02  1.76465e-02  4.33151e-02", "  1.70787e-02  4.23861e-02  1.65642e-02  4.15021e-02  1.60134e-02  4.07315e-02", "  1.53920e-02  4.00690e-02  1.46780e-02  3.93066e-02  1.39739e-02  3.86895e-02", "  1.32306e-02  3.82290e-02  1.23879e-02  3.77215e-02  1.14763e-02  3.73338e-02", "  1.05962e-02  3.70221e-02  9.59117e-03  3.67744e-02  8.55632e-03  3.65904e-02", "  7.54025e-03  3.65357e-02  6.47836e-03  3.66103e-02  5.41058e-03  3.67417e-02", "  4.35776e-03  3.71080e-02  3.11575e-03  3.75625e-02  1.93297e-03  3.81638e-02", "  8.02161e-04  3.89088e-02 -2.68839e-04  3.98709e-02 -1.29221e-03  4.09561e-02", " -2.14878e-03  4.23248e-02 -3.04716e-03  4.39269e-02 -3.55042e-03  4.57788e-02", " -3.98369e-03  4.78259e-02 -3.94844e-03  5.00311e-02 -3.54354e-03  5.22966e-02", " -2.72631e-03  5.46832e-02 -1.45549e-03  5.69609e-02  3.11062e-04  5.90737e-02", "  2.53623e-03  6.08440e-02  5.09003e-03  6.21726e-02  7.84843e-03  6.30819e-02", "  1.07370e-02  6.34527e-02  1.36759e-02  6.32190e-02  1.62666e-02  6.25293e-02", "  1.87388e-02  6.14879e-02  2.10956e-02  6.01686e-02  2.30313e-02  5.85693e-02", "  2.46897e-02  5.67440e-02  2.60303e-02  5.48893e-02  2.71058e-02  5.28327e-02", "  2.80512e-02  5.07326e-02  2.87529e-02  4.85510e-02  2.91959e-02  4.63654e-02", "  2.93466e-02  4.41616e-02  2.93213e-02  4.18216e-02  2.89057e-02  3.92522e-02", "  2.79853e-02  3.67492e-02  2.65890e-02  3.41376e-02  2.43794e-02  3.17572e-02", "  2.13139e-02  2.99079e-02  1.79266e-02  2.92244e-02  1.42512e-02  2.87839e-02", "  8.96759e-03  3.04396e-02  6.37945e-03  3.58098e-02  6.84173e-03  4.02476e-02", "  8.58052e-03  4.36235e-02  1.12738e-02  4.61725e-02  1.49362e-02  4.76295e-02", "  1.93409e-02  4.72653e-02  2.33397e-02  4.45928e-02  2.53093e-02  3.99519e-02", "  2.46466e-02  3.51087e-02  2.20422e-02  3.13247e-02  1.75513e-02  2.88848e-02", "  1.29932e-02  3.35810e-02  1.52743e-02  3.29770e-02  1.39459e-02  3.21647e-02", "  1.25094e-02  3.22451e-02  1.13359e-02  3.27199e-02  1.03082e-02  3.33490e-02", "  9.64984e-03  3.39843e-02  8.96211e-03  3.45373e-02  8.63535e-03  3.51550e-02", "  8.20864e-03  3.56770e-02  7.84962e-03  3.61354e-02  7.45692e-03  3.66037e-02", "  7.01846e-03  3.70839e-02  6.68184e-03  3.75783e-02  6.38937e-03  3.81701e-02", "  5.86698e-03  3.87018e-02  5.48066e-03  3.93657e-02  5.12725e-03  4.00471e-02", "  4.72122e-03  4.09558e-02  4.50711e-03  4.17728e-02  4.25096e-03  4.28344e-02", "  4.04921e-03  4.38827e-02  4.03897e-03  4.50497e-02  4.23696e-03  4.62573e-02", "  4.54588e-03  4.75171e-02  5.04275e-03  4.89675e-02  5.70652e-03  5.02208e-02", "  6.61241e-03  5.14990e-02  7.75804e-03  5.26315e-02  9.09517e-03  5.36392e-02", "  1.06860e-02  5.44909e-02  1.22157e-02  5.50380e-02  1.39103e-02  5.52628e-02", "  1.57251e-02  5.52995e-02  1.73884e-02  5.50176e-02  1.88623e-02  5.45424e-02", "  2.02457e-02  5.38278e-02  2.13367e-02  5.28559e-02  2.23873e-02  5.19359e-02", "  2.31735e-02  5.09295e-02  2.37183e-02  4.99427e-02  2.40718e-02  4.89697e-02", "  2.42779e-02  4.80508e-02  2.43408e-02  4.72015e-02  2.43655e-02  4.64941e-02", "  2.42397e-02  4.58677e-02  2.41610e-02  4.53750e-02  2.38877e-02  4.49717e-02", "  2.37105e-02  4.46712e-02  2.36767e-02  4.45376e-02  2.35923e-02  4.44711e-02", "  2.35944e-02  4.45528e-02  2.36290e-02  4.45581e-02  2.39178e-02  4.46457e-02", "  2.42639e-02  4.47689e-02  2.47544e-02  4.49166e-02  2.54436e-02  4.49153e-02", "  2.62875e-02  4.49566e-02  2.72350e-02  4.46787e-02  2.83833e-02  4.42118e-02", "  2.96985e-02  4.35077e-02  3.10739e-02  4.23099e-02  3.24736e-02  4.05261e-02", "  3.37266e-02  3.79146e-02  3.43720e-02  3.40180e-02  3.33605e-02  2.87081e-02", "  2.83669e-02  2.31747e-02  1.94815e-02  2.23144e-02  1.39923e-02  2.70108e-02", "  1.11951e-02  3.04976e-02  8.78698e-03  3.72408e-02  1.23580e-02  4.19568e-02", "  1.51364e-02  4.33031e-02  1.71239e-02  4.38356e-02  1.85871e-02  4.41430e-02", "  1.97714e-02  4.42862e-02  2.08172e-02  4.43530e-02  2.17973e-02  4.42790e-02", "  2.26572e-02  4.41405e-02  2.33999e-02  4.39398e-02  2.41556e-02  4.37252e-02", "  2.47727e-02  4.34713e-02  2.54252e-02  4.30482e-02  2.58837e-02  4.25068e-02", "  2.63710e-02  4.21697e-02  2.66198e-02  4.17390e-02  2.68731e-02  4.13024e-02", "  2.71007e-02  4.09269e-02  2.72291e-02  4.05107e-02  2.74414e-02  4.01408e-02", "  2.74900e-02  3.98500e-02  2.74907e-02  3.95534e-02  2.75969e-02  3.92282e-02", "  2.76159e-02  3.90443e-02  2.76262e-02  3.88562e-02  2.75761e-02  3.87346e-02", "  2.76604e-02  3.85540e-02  2.76558e-02  3.84981e-02  2.77622e-02  3.83677e-02", "  2.77167e-02  3.84012e-02  2.77313e-02  3.84126e-02  2.78501e-02  3.82973e-02", "  2.79204e-02  3.83297e-02  2.80411e-02  3.83595e-02  2.81818e-02  3.84539e-02", "  2.83580e-02  3.86611e-02  2.85218e-02  3.87534e-02  2.88057e-02  3.88727e-02", "  2.90915e-02  3.90386e-02  2.94567e-02  3.93589e-02  2.99464e-02  3.95274e-02", "  3.04120e-02  3.96769e-02  3.10870e-02  3.98001e-02  3.17770e-02  3.98455e-02", "  3.26659e-02  3.98162e-02  3.35061e-02  3.98174e-02  3.43955e-02  3.95177e-02", "  3.52903e-02  3.90841e-02  3.62019e-02  3.85591e-02  3.71173e-02  3.78621e-02", "  3.78759e-02  3.70448e-02  3.85338e-02  3.63243e-02  3.90189e-02  3.52552e-02", "  3.95050e-02  3.44124e-02  3.98918e-02  3.34746e-02  4.02109e-02  3.24285e-02", "  4.02944e-02  3.14144e-02  4.04481e-02  3.03085e-02  4.05146e-02  2.94549e-02", "  4.04369e-02  2.85059e-02  4.04297e-02  2.75665e-02  4.02063e-02  2.67458e-02", "  4.00836e-02  2.57051e-02  3.98847e-02  2.49267e-02  3.96221e-02  2.39421e-02", "  3.94644e-02  2.31847e-02  3.92243e-02  2.22177e-02  3.88869e-02  2.11931e-02", "  3.85319e-02  2.00665e-02  3.80536e-02  1.89472e-02  3.72941e-02  1.73138e-02", "  3.58921e-02  1.56901e-02  3.37358e-02  1.40264e-02  3.02452e-02  1.30095e-02", "  2.52019e-02  1.48147e-02  2.38516e-02  2.11485e-02  2.90918e-02  2.30423e-02", "  2.83454e-02  1.95815e-02  2.66271e-02  2.23432e-02  2.82972e-02  2.33656e-02", "  2.92692e-02  2.32020e-02  2.98026e-02  2.28301e-02  3.00842e-02  2.24938e-02", "  3.01611e-02  2.21607e-02  3.01884e-02  2.19300e-02  3.01603e-02  2.16103e-02", "  3.01572e-02  2.13756e-02  3.00867e-02  2.11340e-02  2.99885e-02  2.08260e-02", "  2.99162e-02  2.07464e-02  2.98035e-02  2.05434e-02  2.96081e-02  2.03949e-02", "  2.96568e-02  2.02746e-02  2.95706e-02  2.01733e-02  2.95182e-02  2.01072e-02", "  2.94637e-02  1.99284e-02  2.94801e-02  1.97833e-02  2.95564e-02  1.97222e-02", "  2.95823e-02  1.95839e-02  2.97917e-02  1.94753e-02  2.98385e-02  1.93036e-02", "  3.02650e-02  1.90829e-02  3.06539e-02  1.86021e-02  3.12944e-02  1.78823e-02", "  3.17375e-02  1.66142e-02  3.17976e-02  1.51970e-02  3.17343e-02  1.31505e-02", "  3.10034e-02  1.06721e-02  2.89345e-02  7.68720e-03  2.41630e-02  5.39156e-03", "  1.78258e-02  6.12659e-03  1.30761e-02  1.15017e-02  1.31010e-02  1.74219e-02", "  1.49777e-02  2.14957e-02  1.78813e-02  2.36104e-02  2.04205e-02  2.40435e-02", "  2.21093e-02  2.39565e-02  2.34057e-02  2.36773e-02  2.43843e-02  2.32477e-02", "  2.51318e-02  2.28383e-02  2.56008e-02  2.23801e-02  2.59869e-02  2.17986e-02", "  2.62957e-02  2.13528e-02  2.65948e-02  2.10013e-02  2.67341e-02  2.06379e-02", "  2.67196e-02  2.03195e-02  2.68193e-02  2.00674e-02  2.68430e-02  1.98616e-02", "  2.69457e-02  1.96500e-02  2.69126e-02  1.94142e-02  2.68629e-02  1.92576e-02", "  2.70178e-02  1.91495e-02  2.70254e-02  1.89358e-02  2.71410e-02  1.87974e-02", "  2.72527e-02  1.86601e-02  2.73541e-02  1.84922e-02  2.74255e-02  1.83788e-02", "  2.75787e-02  1.81290e-02  2.77451e-02  1.79123e-02  2.79397e-02  1.78154e-02", "  2.79756e-02  1.75721e-02  2.81333e-02  1.72625e-02  2.82057e-02  1.70007e-02", "  2.82682e-02  1.67057e-02  2.82573e-02  1.62809e-02  2.83187e-02  1.60113e-02", "  2.84286e-02  1.57067e-02  2.85517e-02  1.53265e-02  2.84168e-02  1.50471e-02", "  2.83812e-02  1.46137e-02  2.84234e-02  1.42387e-02  2.82636e-02  1.39187e-02", "  2.82694e-02  1.35420e-02  2.81986e-02  1.32026e-02  2.80494e-02  1.29016e-02", "  2.79650e-02  1.25105e-02  2.78312e-02  1.21542e-02  2.76517e-02  1.17449e-02", "  2.74001e-02  1.13679e-02  2.72276e-02  1.11335e-02  2.69776e-02  1.06897e-02", "  2.67285e-02  1.04645e-02  2.64301e-02  1.00683e-02  2.61845e-02  9.76069e-03", "  2.58493e-02  9.56028e-03  2.55609e-02  9.27918e-03  2.53012e-02  9.01256e-03", "  2.50272e-02  8.86128e-03  2.46591e-02  8.66042e-03  2.42905e-02  8.46629e-03", "  2.39279e-02  8.37967e-03  2.36587e-02  8.25170e-03  2.33746e-02  8.14271e-03", "  2.31343e-02  8.01328e-03  2.27966e-02  7.95743e-03  2.26160e-02  7.90013e-03", "  2.23627e-02  7.80513e-03  2.22548e-02  7.73923e-03  2.20662e-02  7.58548e-03", "  2.18058e-02  7.45409e-03  2.16252e-02  7.32496e-03  2.14618e-02  6.99506e-03", "  2.12636e-02  6.90092e-03  2.11518e-02  6.68116e-03  2.07035e-02  6.50971e-03", "  2.06409e-02  6.26130e-03  2.03517e-02  5.97933e-03  2.01118e-02  5.68048e-03", "  1.97292e-02  5.44033e-03  1.93724e-02  5.11140e-03  1.90528e-02  4.79856e-03", "  1.86256e-02  4.63593e-03  1.80995e-02  4.26953e-03  1.76900e-02  4.07323e-03", "  1.71626e-02  3.96314e-03  1.65065e-02  3.77459e-03  1.60554e-02  3.62213e-03", "  1.54624e-02  3.52912e-03  1.48759e-02  3.52004e-03  1.42957e-02  3.49411e-03", "  1.37807e-02  3.54334e-03  1.32063e-02  3.56945e-03  1.25943e-02  3.69636e-03", "  1.22552e-02  3.84885e-03  1.16350e-02  4.02516e-03  1.11906e-02  4.12663e-03", "  1.07385e-02  4.25025e-03  1.01944e-02  4.40194e-03  9.85119e-03  4.61533e-03", "  9.38348e-03  4.84215e-03  9.00230e-03  5.03954e-03  8.64228e-03  5.11429e-03", "  8.30695e-03  5.25426e-03  7.84264e-03  5.57395e-03  7.47936e-03  5.67335e-03", "  7.22287e-03  5.86797e-03  6.76834e-03  6.13320e-03  6.45844e-03  6.22835e-03", "  6.02689e-03  6.43752e-03  5.67707e-03  6.58925e-03  5.27178e-03  6.76587e-03", "  4.77241e-03  6.96632e-03  4.38279e-03  7.27082e-03  3.93170e-03  7.49045e-03", "  3.40365e-03  7.73125e-03  3.01993e-03  7.99480e-03  2.50254e-03  8.37804e-03", "  2.03002e-03  8.79554e-03  1.64412e-03  9.15350e-03  1.20147e-03  9.72035e-03", "  7.72038e-04  1.02086e-02  6.88074e-04  1.07775e-02  8.10250e-04  1.11763e-02", "  9.31347e-04  1.12842e-02  8.17454e-04  1.06564e-02 -7.15987e-04  9.94925e-03", " -2.84202e-03  1.05808e-02 -4.39926e-03  1.24285e-02 -4.82164e-03  1.46462e-02", " -4.61541e-03  1.65040e-02 -3.99818e-03  1.79749e-02 -3.42697e-03  1.89644e-02", " -2.69116e-03  1.98638e-02 -2.15572e-03  2.05507e-02 -1.52530e-03  2.12672e-02", " -9.06652e-04  2.17233e-02 -4.29576e-04  2.21500e-02  3.57893e-04  2.25797e-02", "  9.02656e-04  2.28094e-02  1.46382e-03  2.29983e-02  2.05550e-03  2.30340e-02", "  2.45353e-03  2.30205e-02  2.91697e-03  2.29643e-02  3.29937e-03  2.28135e-02", "  3.50360e-03  2.26948e-02  3.68733e-03  2.25260e-02  3.73264e-03  2.23429e-02", "  3.76445e-03  2.21382e-02  3.67839e-03  2.18742e-02  3.43440e-03  2.18224e-02", "  3.28344e-03  2.16881e-02  2.91442e-03  2.16726e-02  2.60043e-03  2.16708e-02", "  2.19410e-03  2.16683e-02  1.79600e-03  2.18198e-02  1.40477e-03  2.19890e-02", "  9.09325e-04  2.22055e-02  4.03371e-04  2.26217e-02 -6.59255e-06  2.29327e-02", " -5.37596e-04  2.33984e-02 -9.35941e-04  2.41215e-02 -1.46433e-03  2.47107e-02", " -1.93291e-03  2.55763e-02 -2.31742e-03  2.64123e-02 -2.73918e-03  2.71922e-02", " -3.02721e-03  2.83328e-02 -3.17461e-03  2.92938e-02 -3.35304e-03  3.06564e-02", " -3.36692e-03  3.18483e-02 -3.32732e-03  3.32046e-02 -3.11112e-03  3.44822e-02", " -2.64047e-03  3.60578e-02 -2.06282e-03  3.74356e-02 -1.24707e-03  3.89738e-02", " -2.51058e-04  4.03478e-02  8.80202e-04  4.16381e-02  2.31590e-03  4.30584e-02", "  3.75390e-03  4.40515e-02  5.54347e-03  4.50620e-02  7.33913e-03  4.56472e-02", "  9.38228e-03  4.61523e-02  1.14095e-02  4.63472e-02  1.34717e-02  4.63090e-02", "  1.54343e-02  4.60829e-02  1.72383e-02  4.55163e-02  1.90368e-02  4.46497e-02", "  2.06743e-02  4.38244e-02  2.20786e-02  4.27678e-02  2.34145e-02  4.14811e-02", "  2.44666e-02  4.02694e-02  2.53733e-02  3.88998e-02  2.62421e-02  3.76078e-02", "  2.67982e-02  3.62459e-02  2.72438e-02  3.48879e-02  2.76671e-02  3.35706e-02", "  2.77958e-02  3.23074e-02  2.78925e-02  3.09573e-02  2.79382e-02  2.96909e-02", "  2.78980e-02  2.83881e-02  2.77336e-02  2.73571e-02  2.74164e-02  2.61622e-02", "  2.70245e-02  2.50899e-02  2.66643e-02  2.40530e-02  2.61718e-02  2.31239e-02", "  2.56594e-02  2.22053e-02  2.50388e-02  2.14102e-02  2.43752e-02  2.05187e-02", "  2.36109e-02  1.98331e-02  2.27566e-02  1.92185e-02  2.19636e-02  1.86402e-02", "  2.10629e-02  1.81256e-02  2.00472e-02  1.76807e-02  1.92771e-02  1.73994e-02", "  1.81758e-02  1.70641e-02  1.72617e-02  1.69292e-02  1.61690e-02  1.68640e-02", "  1.50589e-02  1.68993e-02  1.39653e-02  1.69989e-02  1.29137e-02  1.72486e-02", "  1.17095e-02  1.77078e-02  1.05487e-02  1.82216e-02  9.29448e-03  1.88895e-02", "  8.35906e-03  1.96828e-02  7.23443e-03  2.07584e-02  6.41200e-03  2.20451e-02", "  5.66931e-03  2.36466e-02  5.16890e-03  2.52345e-02  4.98050e-03  2.72185e-02", "  5.08114e-03  2.92238e-02  5.62788e-03  3.12370e-02  6.67927e-03  3.33762e-02", "  8.11151e-03  3.52690e-02  1.04898e-02  3.68481e-02  1.30174e-02  3.78402e-02", "  1.59141e-02  3.80811e-02  1.90905e-02  3.72873e-02  2.19773e-02  3.53598e-02", "  2.41859e-02  3.27265e-02  2.52967e-02  2.90270e-02  2.51145e-02  2.51331e-02", "  2.32615e-02  2.15132e-02  2.00386e-02  1.86738e-02  1.61703e-02  1.73271e-02", "  1.23975e-02  1.76384e-02  8.90981e-03  1.87827e-02  6.31390e-03  2.07807e-02", "  4.18193e-03  2.31262e-02  2.68295e-03  2.57066e-02  1.73431e-03  2.82425e-02", "  1.14344e-03  3.08800e-02  9.60474e-04  3.37608e-02  1.13549e-03  3.65224e-02", "  1.65667e-03  3.92974e-02  2.62041e-03  4.20368e-02  3.98851e-03  4.48768e-02", "  6.11401e-03  4.74289e-02  8.84592e-03  4.94462e-02  1.16993e-02  5.06436e-02", "  1.46949e-02  5.12892e-02  1.72560e-02  5.14994e-02  1.93912e-02  5.13342e-02", "  2.14080e-02  5.10347e-02  2.32781e-02  5.07361e-02  2.48294e-02  5.04745e-02", "  2.64046e-02  5.03571e-02  2.81330e-02  5.03614e-02  3.02608e-02  4.97702e-02", "  3.20695e-02  4.89353e-02  3.36344e-02  4.83072e-02  3.52932e-02  4.73469e-02", "  3.67551e-02  4.65111e-02  3.82614e-02  4.56314e-02  3.98067e-02  4.44123e-02", "  4.12771e-02  4.31190e-02  4.26072e-02  4.19265e-02  4.39396e-02  4.03175e-02", "  4.51530e-02  3.88120e-02  4.63679e-02  3.69492e-02  4.72938e-02  3.51868e-02", "  4.83230e-02  3.30079e-02  4.91801e-02  3.07005e-02  4.98078e-02  2.82340e-02", "  5.01571e-02  2.50793e-02  5.00004e-02  2.17598e-02  4.89929e-02  1.81674e-02", "  4.68728e-02  1.44337e-02  4.31721e-02  1.16412e-02  3.88336e-02  1.05048e-02", "  3.46822e-02  1.12196e-02  3.24229e-02  1.32309e-02  3.16191e-02  1.41725e-02", "  3.00916e-02  1.41398e-02  2.68831e-02  1.52998e-02  2.56184e-02  1.89722e-02", "  2.66930e-02  2.17583e-02  2.81324e-02  2.29964e-02  2.94033e-02  2.35537e-02", "  3.03557e-02  2.39129e-02  3.12301e-02  2.39378e-02  3.19574e-02  2.38649e-02", "  3.26500e-02  2.38404e-02  3.32956e-02  2.35766e-02  3.38732e-02  2.33879e-02", "  3.42915e-02  2.30504e-02  3.48936e-02  2.26368e-02  3.52760e-02  2.22688e-02", "  3.57471e-02  2.18971e-02  3.63732e-02  2.12564e-02  3.67426e-02  2.08884e-02", "  3.72429e-02  2.02268e-02  3.77023e-02  1.95338e-02  3.81556e-02  1.87573e-02", "  3.87262e-02  1.79002e-02  3.89176e-02  1.69353e-02  3.91923e-02  1.58261e-02", "  3.94085e-02  1.44136e-02  3.95370e-02  1.30634e-02  3.92367e-02  1.17537e-02", "  3.87771e-02  1.02174e-02  3.80862e-02  8.76589e-03  3.71470e-02  7.41860e-03", "  3.58604e-02  6.17182e-03  3.44667e-02  5.15421e-03  3.29222e-02  4.46221e-03", "  3.12477e-02  4.16955e-03  2.97687e-02  4.09294e-03  2.82833e-02  3.97802e-03", "  2.71128e-02  4.51848e-03  2.59246e-02  4.97432e-03  2.48152e-02  5.56863e-03", "  2.39646e-02  6.09851e-03  2.33080e-02  6.73812e-03  2.26684e-02  7.30468e-03", "  2.22482e-02  7.98782e-03  2.18402e-02  8.50778e-03  2.14815e-02  8.94622e-03", "  2.11251e-02  9.43676e-03  2.08505e-02  9.88654e-03  2.06570e-02  1.03898e-02", "  2.04946e-02  1.08227e-02  2.03121e-02  1.13053e-02  2.01923e-02  1.16757e-02", "  2.00767e-02  1.20098e-02  1.98715e-02  1.25967e-02  1.97708e-02  1.30560e-02", "  1.94117e-02  1.36724e-02  1.94718e-02  1.45768e-02  1.98500e-02  1.58343e-02", "  2.14273e-02  1.72835e-02  2.49201e-02  1.63763e-02  2.46298e-02  1.25454e-02", "  2.25601e-02  1.17226e-02  2.13697e-02  1.20315e-02  2.08356e-02  1.23089e-02", "  2.01620e-02  1.23909e-02  1.89490e-02  1.33984e-02  1.94504e-02  1.47639e-02", "  2.07946e-02  1.51813e-02  2.17208e-02  1.38565e-02  2.07739e-02  1.26950e-02", "  1.98596e-02  1.26329e-02  1.90695e-02  1.25634e-02  1.83517e-02  1.23763e-02", "  1.66105e-02  1.24998e-02  1.49661e-02  1.40426e-02  1.45180e-02  1.58125e-02", "  1.46767e-02  1.74359e-02  1.47652e-02  1.87871e-02  1.53209e-02  2.03871e-02", "  1.64091e-02  2.17544e-02  1.79054e-02  2.28083e-02  1.96882e-02  2.33028e-02", "  2.14692e-02  2.31624e-02  2.29828e-02  2.24736e-02  2.41058e-02  2.14185e-02", "  2.47104e-02  2.02619e-02  2.48894e-02  1.91004e-02  2.48366e-02  1.80283e-02", "  2.46923e-02  1.72501e-02  2.41529e-02  1.66325e-02  2.38133e-02  1.59567e-02", "  2.32048e-02  1.57029e-02  2.26688e-02  1.54054e-02  2.22008e-02  1.51784e-02", "  2.16843e-02  1.51595e-02  2.12459e-02  1.50771e-02  2.08133e-02  1.49587e-02", "  2.03503e-02  1.51790e-02  1.98332e-02  1.50612e-02  1.94617e-02  1.52597e-02", "  1.91026e-02  1.55237e-02  1.87231e-02  1.58086e-02  1.83485e-02  1.61461e-02", "  1.79702e-02  1.64893e-02  1.77395e-02  1.67243e-02  1.74502e-02  1.72306e-02", "  1.71691e-02  1.76331e-02  1.69508e-02  1.80034e-02  1.65461e-02  1.84645e-02", "  1.64591e-02  1.90422e-02  1.62855e-02  1.96057e-02  1.62158e-02  2.01641e-02", "  1.61707e-02  2.06612e-02  1.61448e-02  2.15751e-02  1.60944e-02  2.21627e-02", "  1.63539e-02  2.28463e-02  1.66466e-02  2.37310e-02  1.69829e-02  2.44788e-02", "  1.73865e-02  2.51503e-02  1.79723e-02  2.57984e-02  1.86181e-02  2.65077e-02", "  1.93204e-02  2.71029e-02  2.00243e-02  2.76833e-02  2.08501e-02  2.80418e-02", "  2.17405e-02  2.84871e-02  2.26964e-02  2.86013e-02  2.34611e-02  2.87812e-02", "  2.47112e-02  2.87895e-02  2.55013e-02  2.87487e-02  2.62841e-02  2.87852e-02", "  2.73001e-02  2.85711e-02  2.82948e-02  2.80645e-02  2.90129e-02  2.76828e-02", "  2.98323e-02  2.73035e-02  3.05988e-02  2.69290e-02  3.12854e-02  2.62874e-02", "  3.18801e-02  2.58168e-02  3.25784e-02  2.53298e-02  3.30353e-02  2.46126e-02", "  3.35300e-02  2.40743e-02  3.40431e-02  2.34418e-02  3.44209e-02  2.27267e-02", "  3.47835e-02  2.20840e-02  3.52982e-02  2.12425e-02  3.57135e-02  2.05852e-02", "  3.61273e-02  1.96600e-02  3.64366e-02  1.87771e-02  3.68064e-02  1.76148e-02", "  3.71175e-02  1.64691e-02  3.74283e-02  1.50688e-02  3.73521e-02  1.36451e-02", "  3.70994e-02  1.16334e-02  3.61873e-02  9.57782e-03  3.47559e-02  7.49962e-03", "  3.22229e-02  5.92520e-03  2.94800e-02  5.79107e-03  2.71159e-02  6.35825e-03", "  2.51837e-02  7.16506e-03  2.27788e-02  8.47662e-03  2.19707e-02  1.13838e-02", "  2.26524e-02  1.32641e-02  2.35437e-02  1.40393e-02  2.43705e-02  1.44907e-02", "  2.46696e-02  1.46116e-02  2.49908e-02  1.45992e-02  2.53806e-02  1.46233e-02", "  2.54233e-02  1.46890e-02  2.56118e-02  1.46272e-02  2.56541e-02  1.46493e-02", "  2.56401e-02  1.45217e-02  2.56947e-02  1.45144e-02  2.54919e-02  1.44761e-02", "  2.55952e-02  1.44043e-02  2.54303e-02  1.44348e-02  2.53130e-02  1.41289e-02", "  2.51948e-02  1.40960e-02  2.49528e-02  1.40637e-02  2.47767e-02  1.40566e-02", "  2.45968e-02  1.39559e-02  2.44990e-02  1.39343e-02  2.43421e-02  1.38412e-02", "  2.41327e-02  1.40877e-02  2.38662e-02  1.40232e-02  2.36828e-02  1.41866e-02", "  2.33743e-02  1.43913e-02  2.31729e-02  1.44256e-02  2.30785e-02  1.47028e-02", "  2.28061e-02  1.49152e-02  2.27401e-02  1.51163e-02  2.25371e-02  1.53392e-02", "  2.23430e-02  1.55448e-02  2.23991e-02  1.57399e-02  2.22509e-02  1.62108e-02", "  2.22481e-02  1.62654e-02  2.21925e-02  1.65937e-02  2.23868e-02  1.68534e-02", "  2.26326e-02  1.72897e-02  2.26146e-02  1.72423e-02  2.28211e-02  1.75603e-02", "  2.30417e-02  1.77649e-02  2.30635e-02  1.78625e-02  2.33661e-02  1.79139e-02", "  2.36061e-02  1.81098e-02  2.37807e-02  1.81624e-02  2.40343e-02  1.81098e-02", "  2.40557e-02  1.79611e-02  2.42414e-02  1.78652e-02  2.44092e-02  1.77966e-02", "  2.43388e-02  1.77409e-02  2.44193e-02  1.76299e-02  2.45485e-02  1.73549e-02", "  2.44560e-02  1.73657e-02  2.44591e-02  1.74033e-02  2.43533e-02  1.71439e-02", "  2.42349e-02  1.70895e-02  2.41546e-02  1.72335e-02  2.40192e-02  1.72247e-02", "  2.39048e-02  1.71068e-02  2.37896e-02  1.71757e-02  2.36939e-02  1.71343e-02", "  2.35004e-02  1.72429e-02  2.33298e-02  1.73900e-02  2.33010e-02  1.74278e-02", "  2.29971e-02  1.75396e-02  2.29568e-02  1.77088e-02  2.27153e-02  1.78613e-02", "  2.26835e-02  1.80482e-02  2.24490e-02  1.84302e-02  2.22930e-02  1.86599e-02", "  2.22415e-02  1.88938e-02  2.22575e-02  1.93764e-02  2.23083e-02  1.94789e-02", "  2.22685e-02  2.00159e-02  2.22621e-02  2.03216e-02  2.23568e-02  2.06296e-02", "  2.23613e-02  2.10737e-02  2.26383e-02  2.14956e-02  2.27136e-02  2.18806e-02", "  2.28407e-02  2.22036e-02  2.30584e-02  2.24290e-02  2.32231e-02  2.28887e-02", "  2.34429e-02  2.31292e-02  2.37661e-02  2.35169e-02  2.39729e-02  2.38881e-02", "  2.42594e-02  2.41405e-02  2.46088e-02  2.44272e-02  2.49538e-02  2.46282e-02", "  2.52206e-02  2.49328e-02  2.54363e-02  2.51241e-02  2.58769e-02  2.53669e-02", "  2.60835e-02  2.55053e-02  2.64023e-02  2.55496e-02  2.66612e-02  2.58243e-02", "  2.69822e-02  2.62604e-02  2.73495e-02  2.62513e-02  2.76100e-02  2.65394e-02", "  2.80903e-02  2.67536e-02  2.83674e-02  2.69954e-02  2.87406e-02  2.72812e-02", "  2.92413e-02  2.73414e-02  2.96909e-02  2.77490e-02  3.01079e-02  2.79049e-02", "  3.07591e-02  2.82078e-02  3.12651e-02  2.83312e-02  3.17857e-02  2.85068e-02", "  3.23405e-02  2.86673e-02  3.29198e-02  2.89026e-02  3.35621e-02  2.89814e-02", "  3.41157e-02  2.89855e-02  3.48563e-02  2.90098e-02  3.56829e-02  2.91645e-02", "  3.63109e-02  2.90456e-02  3.73135e-02  2.89559e-02  3.80086e-02  2.87217e-02", "  3.88288e-02  2.86073e-02  3.96062e-02  2.82538e-02  4.05061e-02  2.81111e-02", "  4.13849e-02  2.76466e-02  4.22410e-02  2.72362e-02  4.31251e-02  2.66714e-02", "  4.36976e-02  2.60304e-02  4.45097e-02  2.53307e-02  4.52240e-02  2.45495e-02", "  4.57262e-02  2.37685e-02  4.64399e-02  2.28230e-02  4.69992e-02  2.19599e-02", "  4.71882e-02  2.10940e-02  4.77192e-02  2.03587e-02  4.82838e-02  1.91929e-02", "  4.86123e-02  1.80584e-02  4.87243e-02  1.66239e-02  4.89851e-02  1.55113e-02", "  4.90681e-02  1.41451e-02  4.89695e-02  1.26055e-02  4.85511e-02  1.14040e-02", "  4.81367e-02  1.02170e-02  4.75486e-02  8.71139e-03  4.70574e-02  7.53007e-03", "  4.59901e-02  6.24962e-03  4.49437e-02  5.16871e-03  4.39401e-02  4.02697e-03", "  4.26386e-02  3.17416e-03  4.10257e-02  2.39819e-03  3.95213e-02  1.74063e-03", "  3.77057e-02  1.39067e-03  3.57330e-02  1.18766e-03  3.36085e-02  1.43508e-03", "  3.16874e-02  2.33067e-03  2.98928e-02  3.76471e-03  2.88696e-02  5.87441e-03", "  2.95540e-02  7.64761e-03  3.09312e-02  7.31182e-03  3.05614e-02  5.20608e-03", "  2.74257e-02  3.92762e-03  2.36124e-02  4.64462e-03  2.00054e-02  7.41860e-03", "  1.76209e-02  1.14597e-02  1.70059e-02  1.62018e-02  1.75458e-02  2.04045e-02", "  1.87433e-02  2.44683e-02  2.11263e-02  2.86547e-02  2.50411e-02  3.20114e-02", "  2.95829e-02  3.39145e-02  3.42081e-02  3.44893e-02  3.81960e-02  3.36378e-02", "  4.14547e-02  3.20600e-02  4.40418e-02  3.02678e-02  4.57955e-02  2.81722e-02", "  4.73232e-02  2.64914e-02  4.82995e-02  2.42793e-02  4.90826e-02  2.26991e-02", "  4.95402e-02  2.11866e-02  4.96538e-02  1.97134e-02  4.98952e-02  1.84224e-02", "  4.99890e-02  1.70944e-02  4.98373e-02  1.61414e-02  4.96790e-02  1.51796e-02", "  4.96669e-02  1.43243e-02  4.92281e-02  1.35083e-02  4.91749e-02  1.27605e-02", "  4.88975e-02  1.22606e-02  4.86037e-02  1.14756e-02  4.82753e-02  1.12506e-02", "  4.81962e-02  1.06264e-02  4.79147e-02  1.00033e-02  4.76802e-02  9.62882e-03", "  4.74973e-02  9.27923e-03  4.72636e-02  9.06072e-03  4.68814e-02  8.76449e-03", "  4.68247e-02  8.56294e-03  4.66273e-02  8.22679e-03  4.63854e-02  8.21126e-03", "  4.60734e-02  8.13238e-03  4.60723e-02  8.02988e-03  4.60178e-02  7.89963e-03", "  4.58932e-02  7.74516e-03  4.56929e-02  7.85305e-03  4.56731e-02  7.76977e-03", "  4.53854e-02  7.81410e-03  4.55642e-02  7.64167e-03  4.55839e-02  7.69122e-03", "  4.55535e-02  7.59873e-03  4.57899e-02  7.82094e-03  4.58726e-02  7.77015e-03", "  4.59138e-02  7.87533e-03  4.58204e-02  7.82630e-03  4.63974e-02  7.78510e-03", "  4.66728e-02  7.91395e-03  4.68522e-02  7.62795e-03  4.71462e-02  7.57890e-03", "  4.74593e-02  7.59322e-03  4.77858e-02  7.37141e-03  4.81825e-02  7.17835e-03", "  4.84803e-02  6.97346e-03  4.88781e-02  6.67930e-03  4.92272e-02  6.45291e-03", "  4.94642e-02  6.09591e-03  4.99755e-02  5.66019e-03  5.02998e-02  5.37542e-03", "  5.06089e-02  5.00898e-03  5.09089e-02  4.55948e-03  5.11500e-02  3.86054e-03", "  5.14481e-02  3.37818e-03  5.15128e-02  2.77992e-03  5.20474e-02  2.26830e-03", "  5.22084e-02  1.59459e-03  5.24127e-02  9.60249e-04  5.25398e-02  1.71685e-04", "  5.26591e-02 -3.06428e-04  5.28009e-02 -1.14018e-03  5.29360e-02 -1.73446e-03", "  5.28661e-02 -2.37050e-03  5.28378e-02 -3.20237e-03  5.27920e-02 -3.92515e-03", "  5.26408e-02 -4.75771e-03  5.26478e-02 -5.32564e-03  5.25500e-02 -6.20600e-03", "  5.23289e-02 -6.88066e-03  5.23602e-02 -7.56226e-03  5.18177e-02 -8.70348e-03", "  5.16312e-02 -9.64665e-03  5.10020e-02 -1.05462e-02  5.03366e-02 -1.13746e-02", "  5.02518e-02 -1.21732e-02  4.94563e-02 -1.32239e-02  4.86401e-02 -1.39969e-02", "  4.76711e-02 -1.50404e-02  4.68832e-02 -1.58789e-02  4.56011e-02 -1.67246e-02", "  4.41124e-02 -1.78695e-02  4.22334e-02 -1.86517e-02  3.96803e-02 -1.94003e-02", "  3.65699e-02 -1.97206e-02  3.27265e-02 -1.88452e-02  2.80015e-02 -1.63134e-02", "  2.33805e-02 -1.05870e-02  2.36259e-02 -1.38830e-03  3.02833e-02  5.37626e-03", "  3.76351e-02  6.22319e-03  4.26137e-02  4.11255e-03  4.48359e-02  1.88607e-03", "  4.65394e-02 -2.65100e-04  4.72643e-02 -1.80908e-03  4.78687e-02 -3.32670e-03", "  4.82747e-02 -4.33210e-03  4.84320e-02 -5.18053e-03  4.85791e-02 -6.35679e-03", "  4.88728e-02 -7.06833e-03  4.90726e-02 -7.52451e-03  4.93183e-02 -8.43034e-03", "  4.95301e-02 -8.89753e-03  4.98925e-02 -9.56370e-03  5.05409e-02 -1.03931e-02", "  5.09329e-02 -1.09479e-02  5.12285e-02 -1.17898e-02  5.17882e-02 -1.27676e-02", "  5.17893e-02 -1.40817e-02  5.22188e-02 -1.53154e-02  5.21875e-02 -1.62776e-02", "  5.23681e-02 -1.74790e-02  5.21624e-02 -1.85601e-02  5.20607e-02 -1.95450e-02", "  5.19363e-02 -2.08342e-02  5.18329e-02 -2.17593e-02  5.17764e-02 -2.25650e-02", "  5.19902e-02 -2.39153e-02  5.20715e-02 -2.54510e-02  5.17027e-02 -2.75314e-02", "  5.10558e-02 -2.94448e-02  5.03339e-02 -3.06513e-02  4.93782e-02 -3.23453e-02", "  4.83215e-02 -3.37729e-02  4.70582e-02 -3.54946e-02  4.60808e-02 -3.68558e-02", "  4.46219e-02 -3.82386e-02  4.34336e-02 -3.96357e-02  4.16727e-02 -4.09272e-02", "  3.98720e-02 -4.21595e-02  3.78899e-02 -4.37647e-02  3.57306e-02 -4.47090e-02", "  3.35050e-02 -4.56646e-02  3.09986e-02 -4.65331e-02  2.84636e-02 -4.72191e-02", "  2.54009e-02 -4.76717e-02  2.26525e-02 -4.78752e-02  1.92762e-02 -4.76152e-02", "  1.59615e-02 -4.70781e-02  1.25549e-02 -4.60792e-02  9.21533e-03 -4.43239e-02", "  5.98282e-03 -4.21639e-02  2.92166e-03 -3.94145e-02  3.93225e-04 -3.59003e-02", " -1.47679e-03 -3.17197e-02 -2.33638e-03 -2.70735e-02 -2.16465e-03 -2.21087e-02", " -3.01824e-04 -1.74104e-02  3.38857e-03 -1.33905e-02  7.90626e-03 -1.13808e-02", "  1.28573e-02 -1.18003e-02  1.59989e-02 -1.40625e-02  1.72382e-02 -1.67047e-02", "  1.74748e-02 -1.85384e-02  1.81569e-02 -2.00762e-02  1.79019e-02 -2.20937e-02", "  1.70810e-02 -2.37351e-02  1.57417e-02 -2.54532e-02  1.38190e-02 -2.64931e-02", "  1.21859e-02 -2.68828e-02  1.00004e-02 -2.70551e-02  8.28801e-03 -2.66345e-02", "  6.22504e-03 -2.62459e-02  4.62356e-03 -2.54535e-02  3.08416e-03 -2.43005e-02", "  1.77320e-03 -2.34269e-02  5.27639e-04 -2.16650e-02 -3.43972e-04 -2.02337e-02", " -1.32129e-03 -1.87871e-02 -1.98299e-03 -1.74896e-02 -2.27011e-03 -1.56881e-02", " -2.73785e-03 -1.42488e-02 -2.95741e-03 -1.26337e-02 -2.99197e-03 -1.10350e-02", " -2.70485e-03 -9.77767e-03 -2.49600e-03 -8.34802e-03 -2.32046e-03 -7.03889e-03", " -1.92065e-03 -5.75542e-03 -1.38824e-03 -4.58906e-03 -8.83240e-04 -3.57078e-03", " -1.12396e-04 -2.38276e-03  3.16989e-04 -1.60921e-03  1.01726e-03 -3.79637e-04", "  1.48557e-03  3.51247e-04  2.19463e-03  1.03765e-03  3.07952e-03  1.53320e-03", "  3.68215e-03  2.54661e-03  4.54844e-03  2.80469e-03  5.32572e-03  3.40082e-03", "  5.90403e-03  3.93192e-03  6.54690e-03  4.09556e-03  7.44696e-03  4.66296e-03", "  8.10765e-03  4.77052e-03  8.63211e-03  5.34112e-03  9.48479e-03  5.43627e-03", "  1.02591e-02  5.61196e-03  1.07979e-02  6.04656e-03  1.14771e-02  6.16771e-03", "  1.24397e-02  6.52881e-03  1.32303e-02  6.33607e-03  1.37984e-02  6.40683e-03", "  1.46487e-02  6.22952e-03  1.51338e-02  6.34888e-03  1.57010e-02  6.12640e-03", "  1.62515e-02  6.11105e-03  1.68702e-02  5.97189e-03  1.75966e-02  5.51258e-03", "  1.77695e-02  5.27370e-03  1.84239e-02  5.12578e-03  1.86341e-02  4.65444e-03", "  1.90471e-02  4.50552e-03  1.95832e-02  4.11436e-03  1.96386e-02  4.13266e-03", "  1.98161e-02  3.97080e-03  1.98753e-02  3.61232e-03  2.01687e-02  3.56080e-03", "  2.01786e-02  3.37800e-03  2.02422e-02  3.61621e-03  2.03776e-02  3.75073e-03", "  2.07363e-02  4.23985e-03  2.15022e-02  4.64255e-03  2.27969e-02  4.91212e-03", "  2.45981e-02  3.76823e-03  2.57818e-02  2.05777e-03  2.55101e-02 -5.56628e-04", "  2.42072e-02 -2.28315e-03  2.19689e-02 -2.78028e-03  2.11819e-02 -1.69431e-03", "  2.05672e-02 -1.05900e-03  2.02849e-02 -6.93158e-04  2.03760e-02 -3.15899e-04", "  2.06543e-02  2.46952e-04  2.04579e-02  2.09180e-04  2.11113e-02  4.88706e-04", "  2.12365e-02  6.15731e-04  2.12581e-02  6.10635e-04  2.15324e-02  5.42752e-04", "  2.16660e-02  6.40749e-04  2.17656e-02  5.46399e-04  2.20309e-02  4.54312e-04", "  2.17846e-02  3.21583e-04  2.18306e-02  3.01267e-04  2.17891e-02  2.54358e-04", "  2.19372e-02  4.51853e-04  2.18136e-02  2.39841e-04  2.16940e-02  7.40477e-04", "  2.17059e-02  1.31233e-03  2.18586e-02  1.91732e-03  2.22902e-02  2.47737e-03", "  2.32035e-02  2.52373e-03  2.21068e-02  5.33472e-03  2.61430e-02  7.73936e-03", "  3.06137e-02  7.64964e-03  3.56517e-02  4.91334e-03  3.86004e-02  4.22015e-05", "  3.89924e-02 -5.70883e-03  3.70911e-02 -1.05058e-02  3.40995e-02 -1.36998e-02", "  3.07881e-02 -1.57739e-02  2.75601e-02 -1.63911e-02  2.48093e-02 -1.69547e-02", "  2.24038e-02 -1.64232e-02  2.04878e-02 -1.58126e-02  1.88725e-02 -1.49033e-02", "  1.72762e-02 -1.40939e-02  1.63487e-02 -1.32325e-02  1.53677e-02 -1.25099e-02", "  1.45938e-02 -1.14051e-02  1.37568e-02 -1.07488e-02  1.33696e-02 -9.90019e-03", "  1.29122e-02 -8.76190e-03  1.24205e-02 -7.81551e-03  1.23307e-02 -6.80283e-03", "  1.20674e-02 -6.01749e-03  1.22685e-02 -5.30250e-03  1.26331e-02 -4.60606e-03", "  1.26918e-02 -4.11068e-03  1.27763e-02 -3.66205e-03  1.29758e-02 -3.08000e-03", "  1.31268e-02 -2.60402e-03  1.35270e-02 -2.21661e-03  1.36235e-02 -1.98480e-03", "  1.41211e-02 -1.54744e-03  1.41184e-02 -1.19252e-03  1.44485e-02 -1.19342e-03", "  1.47208e-02 -7.23183e-04  1.48242e-02 -4.39667e-04  1.56955e-02 -1.71322e-04", "  1.55696e-02 -5.36243e-05  1.58614e-02 -2.45122e-04  1.61606e-02  2.52086e-05", "  1.61204e-02  1.36252e-04  1.64613e-02 -4.76384e-05  1.66723e-02  1.48229e-04", "  1.69948e-02  2.48437e-04  1.69849e-02  9.17042e-05  1.73122e-02  1.30325e-04", "  1.75075e-02 -9.65372e-07  1.78497e-02  8.11168e-05  1.78725e-02 -6.42235e-05", "  1.83540e-02 -4.13938e-05  1.83959e-02  1.06841e-04  1.85277e-02 -1.70978e-04", "  1.87935e-02  5.43896e-05  1.82604e-02 -3.52411e-04  1.88027e-02 -5.03502e-04", "  1.87276e-02 -2.09943e-04  1.87388e-02 -2.03349e-05  1.90277e-02 -2.12910e-04", "  1.91895e-02 -5.39210e-06  1.93533e-02  2.18422e-04  2.00407e-02 -2.57224e-05", "  2.05178e-02 -2.86896e-04  2.12926e-02 -1.04217e-03  2.14105e-02 -1.93782e-03", "  2.12183e-02 -2.53530e-03  2.08440e-02 -2.98187e-03  2.06870e-02 -3.34448e-03", "  2.06140e-02 -3.47910e-03  2.05676e-02 -3.91937e-03  2.00600e-02 -5.16017e-03", "  1.95283e-02 -5.48827e-03  1.85641e-02 -6.20549e-03  1.73592e-02 -6.46214e-03", "  1.65981e-02 -6.64595e-03  1.49805e-02 -6.12943e-03  1.41132e-02 -5.50807e-03", "  1.36876e-02 -4.52682e-03  1.28674e-02 -3.56184e-03  1.29800e-02 -2.82914e-03", "  1.31238e-02 -1.77943e-03  1.32881e-02 -1.16829e-03  1.34503e-02 -3.50304e-04", "  1.38205e-02 -3.74214e-05  1.42518e-02  3.71544e-04  1.45679e-02  4.84300e-04", "  1.50073e-02  6.27423e-04  1.50724e-02  6.73437e-04  1.56578e-02  8.10832e-04", "  1.56217e-02  6.87128e-04  1.62202e-02  6.04702e-04  1.59606e-02  4.58370e-04", "  1.64204e-02  3.54061e-04  1.64289e-02  7.29181e-05  1.63542e-02 -5.27147e-06", "  1.64335e-02 -4.62007e-04  1.63443e-02 -6.61075e-04  1.62531e-02 -7.86569e-04", "  1.58977e-02 -9.69345e-04  1.56165e-02 -1.36316e-03  1.51241e-02 -1.49868e-03", "  1.45907e-02 -1.37180e-03  1.42929e-02 -1.54945e-03  1.35898e-02 -1.46680e-03", "  1.31385e-02 -9.73406e-04  1.27486e-02 -9.09404e-04  1.24500e-02 -5.52589e-04", "  1.17262e-02  3.65586e-06  1.16288e-02  2.70840e-04  1.15826e-02  8.21275e-04", "  1.15413e-02  1.10288e-03  1.11549e-02  1.34318e-03  1.13853e-02  2.10586e-03", "  1.14195e-02  2.29532e-03  1.15468e-02  2.89524e-03  1.11639e-02  3.06574e-03", "  1.13769e-02  3.26006e-03  1.11099e-02  3.84802e-03  1.13097e-02  4.13241e-03", "  1.14750e-02  4.57083e-03  1.14298e-02  4.68863e-03  1.13664e-02  4.83929e-03", "  1.12927e-02  5.35525e-03  1.15434e-02  5.67112e-03  1.15159e-02  5.88725e-03", "  1.17264e-02  6.08231e-03  1.16440e-02  6.56969e-03  1.16579e-02  6.67163e-03", "  1.19027e-02  6.94171e-03  1.20091e-02  7.17963e-03  1.18900e-02  7.40229e-03", "  1.20231e-02  7.60731e-03  1.22161e-02  7.82924e-03  1.24377e-02  7.97899e-03", "  1.25161e-02  8.22324e-03  1.23675e-02  8.49602e-03  1.27115e-02  8.40710e-03", "  1.25652e-02  8.98065e-03  1.28820e-02  9.13251e-03  1.28883e-02  9.15257e-03", "  1.30471e-02  9.55393e-03  1.29672e-02  9.77988e-03  1.31733e-02  1.02340e-02", "  1.31457e-02  1.01378e-02  1.33051e-02  1.05134e-02  1.35002e-02  1.09118e-02", "  1.33473e-02  1.11494e-02  1.33813e-02  1.10995e-02  1.34339e-02  1.12686e-02", "  1.34938e-02  1.15099e-02  1.38657e-02  1.17962e-02  1.36997e-02  1.21476e-02", "  1.38315e-02  1.21688e-02  1.41581e-02  1.27145e-02  1.40726e-02  1.27922e-02", "  1.42246e-02  1.31773e-02  1.42663e-02  1.36986e-02  1.41527e-02  1.39200e-02", "  1.39579e-02  1.43339e-02  1.43741e-02  1.44867e-02  1.42167e-02  1.49198e-02", "  1.44147e-02  1.53428e-02  1.43108e-02  1.57935e-02  1.43382e-02  1.63784e-02", "  1.44033e-02  1.68239e-02  1.46771e-02  1.72616e-02  1.46100e-02  1.80015e-02", "  1.47750e-02  1.87190e-02  1.47207e-02  1.89364e-02  1.51937e-02  1.98903e-02", "  1.50938e-02  2.03018e-02  1.52822e-02  2.09539e-02  1.58685e-02  2.16663e-02", "  1.58973e-02  2.24557e-02  1.63441e-02  2.32572e-02  1.67721e-02  2.41730e-02", "  1.72586e-02  2.49277e-02  1.80120e-02  2.56028e-02  1.84600e-02  2.66718e-02", "  1.94745e-02  2.73299e-02  2.01435e-02  2.82443e-02  2.07326e-02  2.93102e-02", "  2.21816e-02  3.00045e-02  2.31823e-02  3.05428e-02  2.44421e-02  3.12073e-02", "  2.61684e-02  3.18911e-02  2.76073e-02  3.20029e-02  2.93875e-02  3.20064e-02", "  3.14520e-02  3.19444e-02  3.32965e-02  3.14716e-02  3.51009e-02  2.98206e-02", "  3.67658e-02  2.77609e-02  3.71376e-02  2.48218e-02  3.59205e-02  2.07904e-02", "  3.14570e-02  1.84531e-02  2.51758e-02  2.03932e-02  2.18135e-02  2.73516e-02", "  2.46236e-02  3.28898e-02  2.73845e-02  3.49376e-02  2.93101e-02  3.73294e-02", "  3.30638e-02  3.97111e-02  3.73131e-02  4.09389e-02  4.12062e-02  3.98505e-02", "  4.47363e-02  3.84259e-02  4.75320e-02  3.66169e-02  4.94683e-02  3.42082e-02", "  5.11579e-02  3.12037e-02  5.15270e-02  2.87462e-02  5.05773e-02  2.65862e-02", "  4.97301e-02  2.57128e-02  4.87497e-02  2.54978e-02  4.92227e-02  2.63027e-02", "  5.06317e-02  2.68939e-02  5.22746e-02  2.49646e-02  5.23741e-02  2.32009e-02", "  5.06187e-02  2.14855e-02  4.96530e-02  2.20260e-02  4.97771e-02  2.35157e-02", "  5.12276e-02  2.34033e-02  5.24913e-02  2.24650e-02  5.22107e-02  2.11277e-02", "  5.13576e-02  2.01451e-02  5.05437e-02  1.99535e-02  4.92713e-02  2.12792e-02", "  4.84541e-02  2.28533e-02  4.92848e-02  2.52313e-02  5.08506e-02  2.64206e-02", "  5.27325e-02  2.75024e-02  5.41227e-02  2.82030e-02  5.53815e-02  2.92884e-02", "  5.70516e-02  3.08838e-02  6.01860e-02  3.26765e-02  6.44561e-02  3.32596e-02", "  6.85108e-02  3.24690e-02  7.30698e-02  3.06881e-02  7.61377e-02  2.81878e-02", "  7.87030e-02  2.48313e-02  8.06554e-02  2.14048e-02  8.20955e-02  1.84304e-02", "  8.27474e-02  1.51599e-02  8.27798e-02  1.22525e-02  8.28403e-02  9.56228e-03", "  8.34897e-02  6.93129e-03  8.28073e-02  4.95435e-03  8.28431e-02  2.67034e-03", "  8.21577e-02  8.12907e-04  8.18441e-02 -1.15346e-03  8.12870e-02 -2.70351e-03", "  8.05612e-02 -4.16358e-03  8.04340e-02 -5.54137e-03  7.98544e-02 -6.67202e-03", "  7.88474e-02 -8.02757e-03  7.85452e-02 -9.54907e-03  7.76535e-02 -1.05584e-02", "  7.72766e-02 -1.12042e-02  7.67704e-02 -1.21568e-02  7.63134e-02 -1.31358e-02", "  7.55638e-02 -1.44061e-02  7.55250e-02 -1.48399e-02  7.49403e-02 -1.57260e-02", "  7.47116e-02 -1.61729e-02  7.43480e-02 -1.70748e-02  7.41898e-02 -1.79178e-02", "  7.37389e-02 -1.82010e-02  7.36314e-02 -1.92747e-02  7.31360e-02 -1.97923e-02", "  7.25300e-02 -2.02911e-02  7.21967e-02 -2.13057e-02  7.20872e-02 -2.23671e-02", "  7.18715e-02 -2.31776e-02  7.15837e-02 -2.39951e-02  7.12092e-02 -2.43844e-02", "  7.06233e-02 -2.49788e-02  7.02366e-02 -2.57398e-02  6.99790e-02 -2.64932e-02", "  6.99655e-02 -2.66890e-02  6.93542e-02 -2.76534e-02  6.92545e-02 -2.83192e-02", "  6.91439e-02 -2.91609e-02  6.87283e-02 -2.94965e-02  6.86269e-02 -3.01281e-02", "  6.85993e-02 -3.09026e-02  6.79883e-02 -3.17333e-02  6.81935e-02 -3.28104e-02", "  6.73275e-02 -3.33404e-02  6.75497e-02 -3.39908e-02  6.72486e-02 -3.47384e-02", "  6.68608e-02 -3.58155e-02  6.61874e-02 -3.70489e-02  6.63411e-02 -3.74338e-02", "  6.61303e-02 -3.82590e-02  6.54675e-02 -3.89058e-02  6.49813e-02 -4.01246e-02", "  6.48547e-02 -4.13160e-02  6.39181e-02 -4.19805e-02  6.36322e-02 -4.30607e-02", "  6.34624e-02 -4.38713e-02  6.24205e-02 -4.48627e-02  6.16028e-02 -4.52513e-02", "  6.09744e-02 -4.68421e-02  6.04347e-02 -4.71731e-02  5.99663e-02 -4.81012e-02", "  5.87509e-02 -4.92601e-02  5.85174e-02 -4.97230e-02  5.73570e-02 -5.08442e-02", "  5.67581e-02 -5.12154e-02  5.55768e-02 -5.22153e-02  5.43458e-02 -5.30419e-02", "  5.36812e-02 -5.33041e-02  5.28445e-02 -5.39367e-02  5.16232e-02 -5.50334e-02", "  5.12313e-02 -5.58829e-02  4.96159e-02 -5.64434e-02  4.89605e-02 -5.67812e-02", "  4.71896e-02 -5.71987e-02  4.66558e-02 -5.77128e-02  4.49551e-02 -5.81017e-02", "  4.41132e-02 -5.83516e-02  4.34710e-02 -5.90885e-02  4.23098e-02 -5.93960e-02", "  4.06641e-02 -5.95332e-02  3.95444e-02 -5.97470e-02  3.84398e-02 -5.97979e-02", "  3.78106e-02 -6.05267e-02  3.66654e-02 -5.99958e-02  3.54147e-02 -6.00916e-02", "  3.44865e-02 -6.03344e-02  3.33624e-02 -6.06445e-02  3.24358e-02 -6.02802e-02", "  3.15447e-02 -6.02360e-02  3.05874e-02 -6.04049e-02  2.99556e-02 -6.02936e-02", "  2.82405e-02 -6.04908e-02  2.75224e-02 -6.06318e-02  2.68085e-02 -6.06954e-02", "  2.59640e-02 -6.06211e-02  2.49166e-02 -6.08111e-02  2.37318e-02 -6.08362e-02", "  2.27860e-02 -6.04672e-02  2.16407e-02 -6.06607e-02  2.07520e-02 -6.05305e-02", "  1.94305e-02 -6.00309e-02  1.87765e-02 -5.95611e-02  1.72486e-02 -6.00756e-02", "  1.63012e-02 -5.95605e-02  1.51288e-02 -5.93870e-02  1.41173e-02 -5.88064e-02", "  1.34366e-02 -5.86788e-02  1.20626e-02 -5.79885e-02  1.12956e-02 -5.82534e-02", "  1.03307e-02 -5.74751e-02  9.29928e-03 -5.69908e-02  8.52216e-03 -5.65608e-02", "  7.75912e-03 -5.58800e-02  6.61906e-03 -5.45576e-02  6.05627e-03 -5.42466e-02", "  5.28230e-03 -5.36570e-02  4.48353e-03 -5.28966e-02  4.05670e-03 -5.23036e-02", "  3.38102e-03 -5.20194e-02  2.78441e-03 -5.10949e-02  1.86215e-03 -5.06088e-02", "  1.07778e-03 -5.00262e-02  7.53056e-04 -4.90585e-02 -1.82193e-04 -4.86814e-02", " -4.55253e-04 -4.79546e-02 -1.42491e-03 -4.71701e-02 -1.80490e-03 -4.64212e-02", " -2.15924e-03 -4.56165e-02 -3.00334e-03 -4.50226e-02 -3.62015e-03 -4.41052e-02", " -4.92322e-03 -4.32834e-02 -5.32097e-03 -4.24233e-02 -5.95635e-03 -4.14979e-02", " -6.32222e-03 -4.07013e-02 -6.92096e-03 -3.95761e-02 -7.29955e-03 -3.86260e-02", " -7.79575e-03 -3.73299e-02 -8.21415e-03 -3.58706e-02 -8.57541e-03 -3.48052e-02", " -8.95907e-03 -3.32147e-02 -8.71960e-03 -3.17776e-02 -9.24992e-03 -3.03379e-02", " -9.01035e-03 -2.87945e-02 -8.50274e-03 -2.71686e-02 -8.25240e-03 -2.56415e-02", " -7.71980e-03 -2.37485e-02 -6.74245e-03 -2.25745e-02 -5.33137e-03 -2.15223e-02", " -4.01202e-03 -2.08864e-02 -2.60352e-03 -1.99786e-02 -1.63921e-03 -2.00599e-02", " -2.95759e-04 -1.98609e-02  4.11462e-04 -1.95718e-02  1.42077e-03 -1.91953e-02", "  2.55944e-03 -1.96548e-02  3.54886e-03 -1.93092e-02  4.28443e-03 -2.00448e-02", "  4.64587e-03 -2.13377e-02  5.69941e-03 -2.15123e-02  5.48284e-03 -2.26262e-02", "  5.40093e-03 -2.31540e-02  5.32559e-03 -2.39386e-02  4.64419e-03 -2.43989e-02", "  3.96804e-03 -2.49642e-02  3.17888e-03 -2.51684e-02  2.44880e-03 -2.50980e-02", "  1.30922e-03 -2.52208e-02  1.27570e-03 -2.39239e-02  1.14088e-04 -2.40974e-02", " -8.49384e-05 -2.33928e-02 -5.73352e-04 -2.23807e-02 -1.00177e-03 -2.15384e-02", " -8.31305e-04 -2.08770e-02 -7.85251e-04 -2.03822e-02 -1.36371e-04 -1.91298e-02", " -4.27699e-06 -1.85301e-02  1.30764e-04 -1.79877e-02  7.94438e-04 -1.74426e-02", "  1.28578e-03 -1.68225e-02  1.62590e-03 -1.66115e-02  1.58471e-03 -1.64615e-02", "  2.08581e-03 -1.58438e-02  2.42584e-03 -1.58921e-02  3.11916e-03 -1.56913e-02", "  3.41748e-03 -1.57830e-02  3.66909e-03 -1.55621e-02  3.51624e-03 -1.57982e-02", "  4.13079e-03 -1.54612e-02  4.34436e-03 -1.57606e-02  4.33127e-03 -1.56684e-02", "  4.65317e-03 -1.51794e-02  5.19616e-03 -1.49783e-02  5.27430e-03 -1.53630e-02", "  5.36732e-03 -1.49836e-02  5.15634e-03 -1.55162e-02  5.31412e-03 -1.52685e-02", "  5.47407e-03 -1.52107e-02  5.67977e-03 -1.49730e-02  5.56688e-03 -1.47417e-02", "  5.75291e-03 -1.45563e-02  6.01333e-03 -1.43341e-02  5.79255e-03 -1.40530e-02", "  5.50785e-03 -1.37779e-02  6.20327e-03 -1.40307e-02  6.15748e-03 -1.32341e-02", "  6.59303e-03 -1.28854e-02  6.53045e-03 -1.25725e-02  7.14529e-03 -1.23956e-02", "  7.20081e-03 -1.21964e-02  8.27579e-03 -1.17768e-02  9.07314e-03 -1.15471e-02", "  9.34503e-03 -1.18018e-02  1.04765e-02 -1.17051e-02  1.16417e-02 -1.22968e-02", "  1.12376e-02 -1.29724e-02  1.12567e-02 -1.40361e-02  1.09181e-02 -1.42788e-02", "  1.04482e-02 -1.45766e-02  9.67280e-03 -1.43913e-02  9.83214e-03 -1.40303e-02", "  9.90929e-03 -1.34447e-02  1.03061e-02 -1.36042e-02  1.07517e-02 -1.28885e-02", "  1.08869e-02 -1.33497e-02  1.08050e-02 -1.35827e-02  1.13636e-02 -1.30864e-02", "  1.15344e-02 -1.25292e-02  1.18106e-02 -1.27665e-02  1.20030e-02 -1.30864e-02", "  1.19970e-02 -1.30285e-02  1.19134e-02 -1.28052e-02  1.17019e-02 -1.32553e-02", "  1.25983e-02 -1.27920e-02  1.26044e-02 -1.30025e-02  1.28679e-02 -1.32016e-02", "  1.31488e-02 -1.29549e-02  1.32888e-02 -1.29386e-02  1.39612e-02 -1.33676e-02", "  1.38369e-02 -1.32241e-02  1.40315e-02 -1.30660e-02  1.41936e-02 -1.33438e-02", "  1.49349e-02 -1.34628e-02  1.54483e-02 -1.32503e-02  1.53208e-02 -1.39360e-02", "  1.59246e-02 -1.43186e-02  1.53275e-02 -1.43150e-02  1.58723e-02 -1.44503e-02", "  1.54020e-02 -1.51246e-02  1.58178e-02 -1.46506e-02  1.58864e-02 -1.50152e-02", "  1.62523e-02 -1.52916e-02  1.61714e-02 -1.57184e-02  1.60745e-02 -1.60996e-02", "  1.57931e-02 -1.62538e-02  1.65964e-02 -1.62220e-02  1.56430e-02 -1.65480e-02", "  1.62939e-02 -1.70254e-02  1.55967e-02 -1.72464e-02  1.62961e-02 -1.76523e-02", "  1.58506e-02 -1.76287e-02  1.61035e-02 -1.76577e-02  1.55062e-02 -1.82831e-02", "  1.53987e-02 -1.82794e-02  1.55587e-02 -1.83272e-02  1.50845e-02 -1.90579e-02", "  1.50012e-02 -1.90982e-02  1.48210e-02 -1.90622e-02  1.44754e-02 -1.95290e-02", "  1.49211e-02 -1.96494e-02  1.42352e-02 -2.00033e-02  1.42929e-02 -2.02494e-02", "  1.34255e-02 -2.03010e-02  1.33455e-02 -2.02058e-02  1.33529e-02 -2.06962e-02", "  1.29853e-02 -2.05738e-02  1.28878e-02 -2.06592e-02  1.23345e-02 -2.12358e-02", "  1.23759e-02 -2.10484e-02  1.13238e-02 -2.06836e-02  1.13520e-02 -2.09309e-02", "  1.03990e-02 -2.08252e-02  1.05220e-02 -2.18437e-02  8.25291e-03 -2.14335e-02", "  5.24270e-03 -1.95948e-02  5.78224e-03 -1.48500e-02  9.27599e-03 -1.19439e-02", "  1.50797e-02 -1.32328e-02  1.60219e-02 -1.81737e-02  1.42985e-02 -2.05687e-02", "  1.28581e-02 -2.18695e-02  1.17549e-02 -2.11582e-02  1.10393e-02 -2.12846e-02", "  1.08025e-02 -2.13900e-02  1.02844e-02 -2.07286e-02  9.78147e-03 -2.08050e-02", "  9.27868e-03 -2.07936e-02  8.94692e-03 -2.04946e-02  9.14603e-03 -2.03235e-02", "  8.08488e-03 -2.07061e-02  7.67966e-03 -2.01124e-02  7.52155e-03 -2.04056e-02", "  7.55710e-03 -2.02195e-02  6.70879e-03 -1.99507e-02  6.56623e-03 -1.96176e-02", "  5.53982e-03 -2.00755e-02  5.58106e-03 -1.96831e-02  4.67393e-03 -1.90585e-02", "  3.81889e-03 -1.79193e-02  3.67888e-03 -1.75198e-02  2.79013e-03 -1.63333e-02", "  2.21188e-03 -1.50357e-02  2.63350e-03 -1.38755e-02  2.93824e-03 -1.30897e-02", "  3.19720e-03 -1.19090e-02  3.42754e-03 -1.08108e-02  4.36852e-03 -9.88622e-03", "  4.91314e-03 -9.34348e-03  6.07306e-03 -8.75742e-03  6.90491e-03 -8.32568e-03", "  7.46031e-03 -7.77528e-03  8.26481e-03 -7.51107e-03  9.24431e-03 -6.88049e-03", "  9.91556e-03 -6.41822e-03  1.09484e-02 -5.98616e-03  1.14118e-02 -6.05355e-03", "  1.21809e-02 -6.24608e-03  1.26498e-02 -6.65211e-03  1.32222e-02 -6.15536e-03", "  1.46351e-02 -6.69838e-03  1.51935e-02 -7.24355e-03  1.56745e-02 -7.21952e-03", "  1.66043e-02 -6.93911e-03  1.68295e-02 -7.31034e-03  1.79383e-02 -8.00691e-03", "  1.78996e-02 -8.20326e-03  1.83711e-02 -8.58486e-03  1.90073e-02 -8.90909e-03", "  1.93850e-02 -8.78277e-03  1.99077e-02 -9.66427e-03  1.96080e-02 -1.00428e-02", "  2.05043e-02 -1.04842e-02  2.06335e-02 -1.09816e-02", ""]) -> (3 "DataSet":T1={"Abscissa"={"Specific Data Type"=enum."Unknown", "Length unit exponent"=0, "Force units exponent"=0, "Temperature unit exponent"=0, "Axis Label"="Frequency", "Axis Label Unit"="Hz"}, "Ordinate Numerator"={"Specific Data Type"=enum."Unknown", "Length unit exponent"=0, "Force units exponent"=0, "Temperature unit exponent"=0, "Axis Label"="Velocity", "Axis Label Unit"="m/s"}, "Ordinate Denominator"={"Specific Data Type"=enum."Unknown", "Length unit exponent"=0, "Force units exponent"=0, "Temperature unit exponent"=0, "Axis Label"="Force", "Axis Label Unit"="N"}, "Z Axis"={"Specific Data Type"=enum."Unknown", "Length unit exponent"=0, "Force units exponent"=0, "Temperature unit exponent"=0, "Axis Label"="NONE", "Axis Label Unit"="NONE"}, "Data Form"={"Ordinate Data Type"=enum."NA", "# values or pairs"=3200, "Abscissa Spacing"=enum."Uneven", "Abscissa min"=1.25, "Abscissa inc"=1.25, "Z Axis Value"=0.0}, "DOF ID"={"Function Type"=enum."General or Unknown", "Function ID #"=3, "Version Number"=1, "Load Case ID"=enum."Single Point Excitation", "Response Name"="NONE", "Response Node"=513, "Response Direction"=0, "Reference Name"="NONE", "Reference Node"=501, "Reference Direction"=0}, "Data"={0.0, 0.0, []}, "Header"=""} {"DOF ID"."Reference Direction" items=["-Z Rotation"=-6, "-Y Rotation"=-5, "-X Rotation"=-4, "-Z Translation"=-3, "-Y Translation"=-2, "-X Translation"=-1, "Scalar"=0, "X Translaation"=1, "Y Translation"=2, "Z Translation"=3, "X Rotation"=4, "Y Rotation"=5, "Z Rotation"=6]; "DOF ID"."Response Direction" items=["-Z Rotation"=-6, "-Y Rotation"=-5, "-X Rotation"=-4, "-Z Translation"=-3, "-Y Translation"=-2, "-X Translation"=-1, "Scalar"=0, "X Translaation"=1, "Y Translation"=2, "Z Translation"=3, "X Rotation"=4, "Y Rotation"=5, "Z Rotation"=6]})   [LabVIEW 2022 SP3]
uses:
  <vilib>/Utility/error.llb/Trim Whitespace One-Sided.vi
panel:
  out "size(s)":i32
  out "UF Dataset type":i32=58
  # "values for even spacing\npairs for uneven spacing"
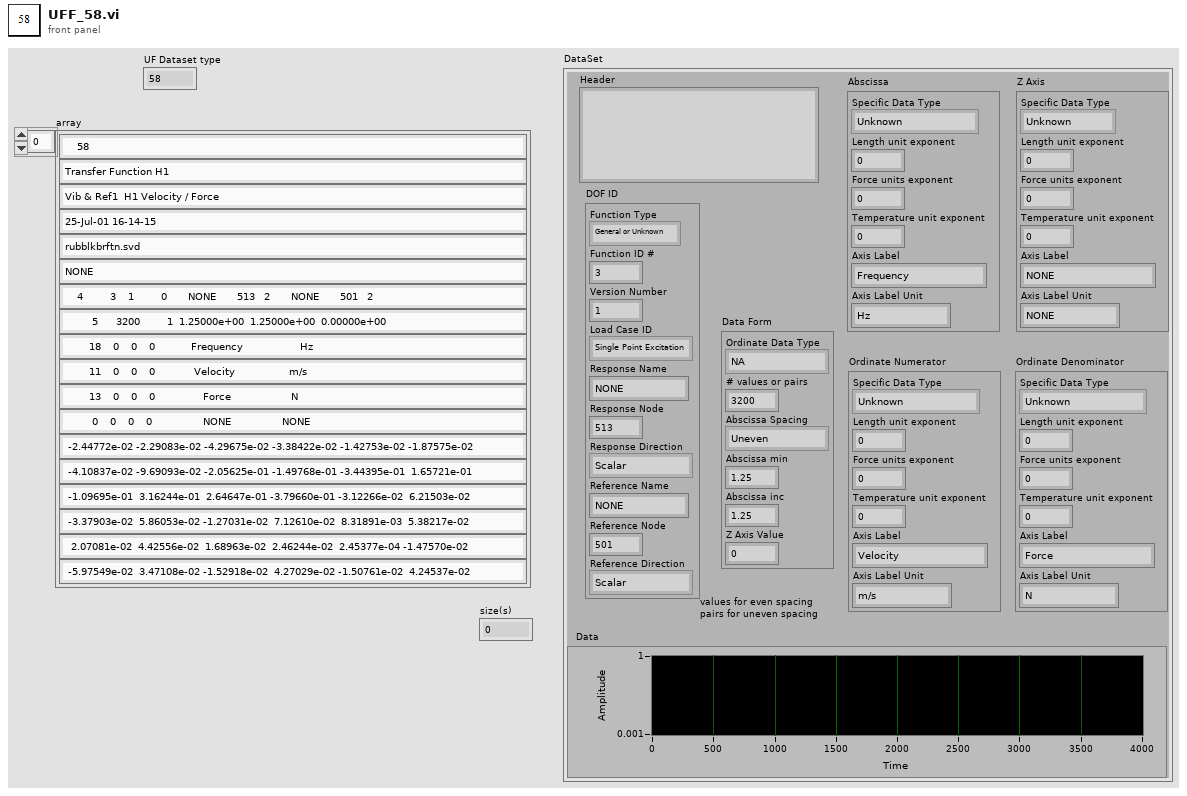
[diagram p1: front panel]
types:
  T1 = cluster{"Abscissa":cluster{"Specific Data Type":enum16{"Unknown", "general", "stress", "strain", "na1", "temperature", "heat flux", "displacement", "na2", "reaction force", "na3", "velocity", "acceleration", "excitation force", "na4", "pressure", "mass", "time", "frequency", "rpm", "order", "sound pressure", "sound intensity", "sound power"}, "Length unit exponent":i32, "Force units exponent":i32, "Temperature unit exponent":i32, "Axis Label":string, "Axis Label Unit":string}, "Ordinate Numerator":cluster{"Specific Data Type":enum16{"Unknown", "general", "stress", "strain", "na1", "temperature", "heat flux", "displacement", "na2", "reaction force", "na3", "velocity", "acceleration", "excitation force", "na4", "pressure", "mass", "time", "frequency", "rpm", "order", "sound pressure", "sound intensity", "sound power"}, "Length unit exponent":i32, "Force units exponent":i32, "Temperature unit exponent":i32, "Axis Label":string, "Axis Label Unit":string}, "Ordinate Denominator":cluster{"Specific Data Type":enum16{"Unknown", "general", "stress", "strain", "na1", "temperature", "heat flux", "displacement", "na2", "reaction force", "na3", "velocity", "acceleration", "excitation force", "na4", "pressure", "mass", "time", "frequency", "rpm", "order", "sound pressure", "sound intensity", "sound power"}, "Length unit exponent":i32, "Force units exponent":i32, "Temperature unit exponent":i32, "Axis Label":string, "Axis Label Unit":string}, "Z Axis":cluster{"Specific Data Type":enum16{"Unknown", "general", "stress", "strain", "na1", "temperature", "heat flux", "displacement", "na2", "reaction force", "na3", "velocity", "acceleration", "excitation force", "na4", "pressure", "mass", "time", "frequency", "rpm", "order", "sound pressure", "sound intensity", "sound power"}, "Length unit exponent":i32, "Force units exponent":i32, "Temperature unit exponent":i32, "Axis Label":string, "Axis Label Unit":string}, "Data Form":cluster{"Ordinate Data Type":enum16{"NA", "NA2", "Real SGL", "NA3", "Real DBL", "Complex SGL", "Complex DBL"}, "# values or pairs":i32, "Abscissa Spacing":enum16{"Uneven", "Even"}, "Abscissa min":dbl, "Abscissa inc":dbl, "Z Axis Value":dbl}, "DOF ID":cluster{"Function Type":enum16{"General or Unknown", "Time Response", "Auto Spectrum", "Cross Spectrum", "FRF", "Transmissibility", "Coherence", "Auto Correlation", "Cross Correlation", "Power Spectral Density", "Energy Spectral Density Function", "Prob Density Function", "Spectrum", "Cumulative Freq Dist", "Peaks Valley", "Stress/Cycles", "Strain/Cycles", "Orbit", "Mode Indicator Funct", "Force Pattern", "Partial Power", "Partial Coherence", "Eigenvalue", "Eigenvector", "Shock Response Spectrum", "Finite Inpulse Response Filter", "Multiple Coherence", "Order Function", "Phase Compensation"}, "Function ID #":i32, "Version Number":i32, "Load Case ID":enum16{"Single Point Excitation"}, "Response Name":string, "Response Node":i32, "Response Direction":i8, "Reference Name":string, "Reference Node":i32, "Reference Direction":i8}, "Data":cluster{dbl, dbl, dbl[]}, "Header":string}
  T2 = enum16{"NA", "NA2", "Real SGL", "NA3", "Real DBL", "Complex SGL", "Complex DBL"}
  T3 = cluster{"Value":i32, "Value":i32, "Value":i32, "Value":i32, "Subset":string, "Value":i32, "Value":i32, "Subset":string, "Value":i32, "Value":i32}
  T4 = cluster{"Value":i32, "Value":i32, "Value":i32, "number":dbl, "number":dbl, "number":dbl}
  T5 = cluster{"Value":i32, "Value":i32, "Value":i32, "Value":i32, "Subset":string, "Subset":string}
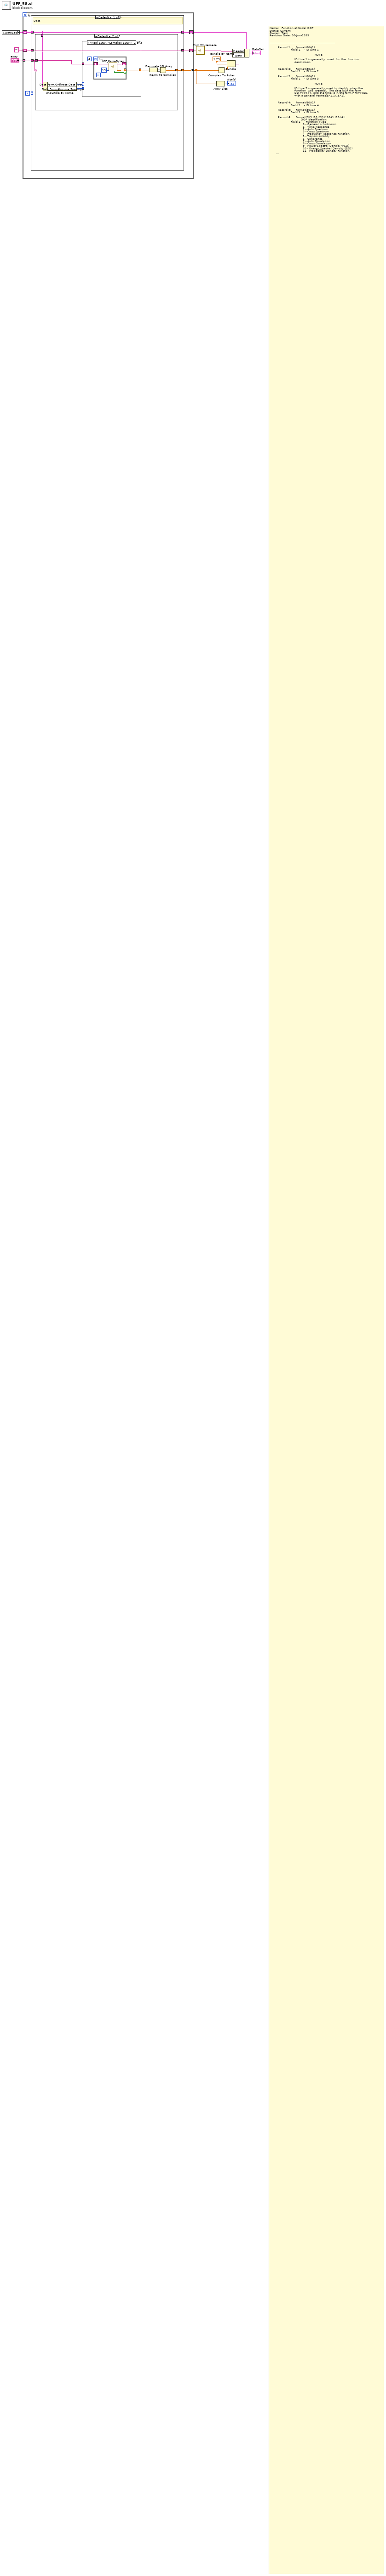
[diagram p0: block diagram]
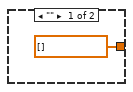
[diagram p2: hidden frame]
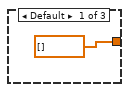
[diagram p3: hidden frame]
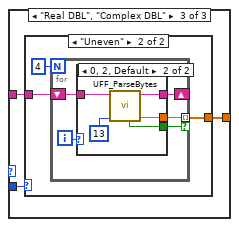
[diagram p4: hidden frame]
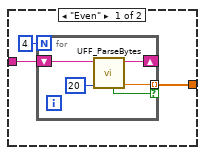
[diagram p5: hidden frame]
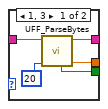
[diagram p6: hidden frame]
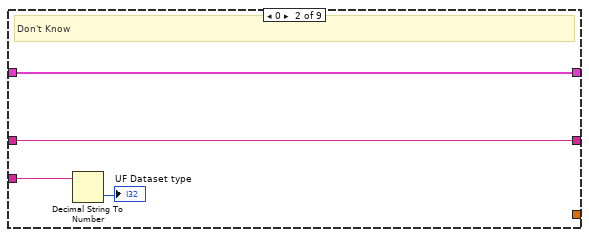
[diagram p7: hidden frame]
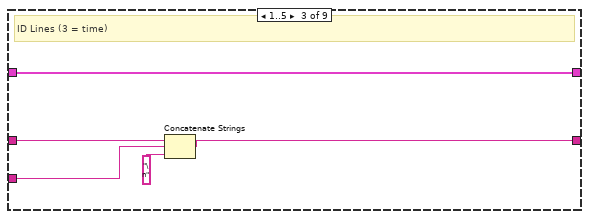
[diagram p8: hidden frame]
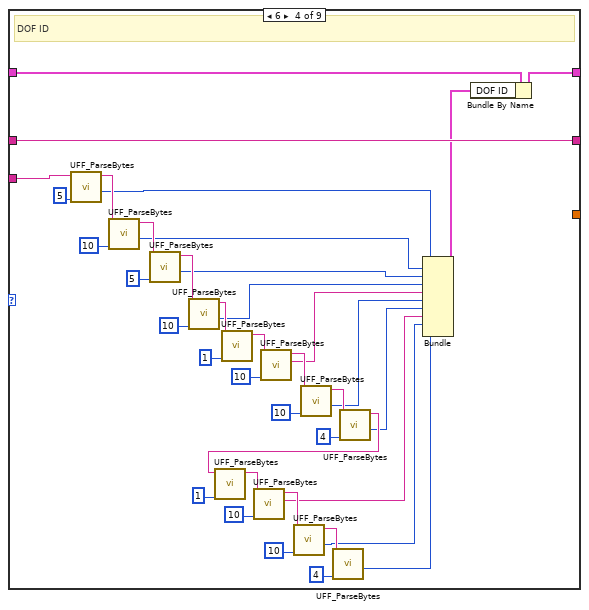
[diagram p9: hidden frame]
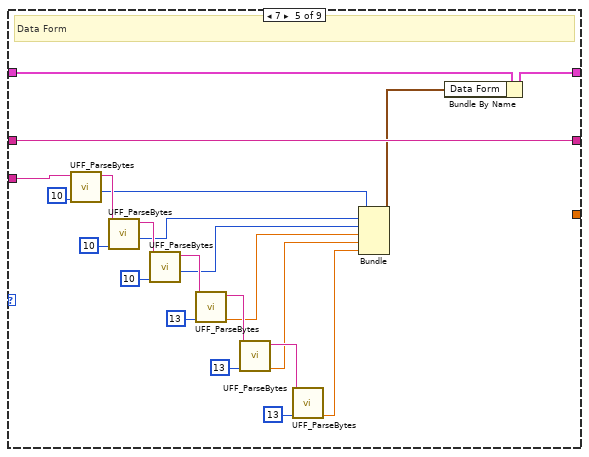
[diagram p10: hidden frame]
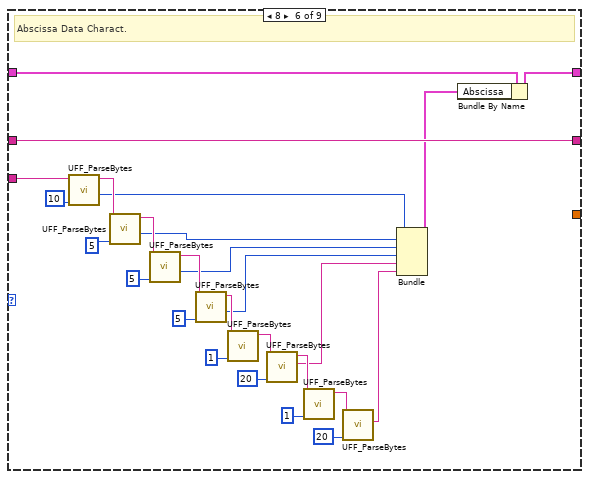
[diagram p11: hidden frame]
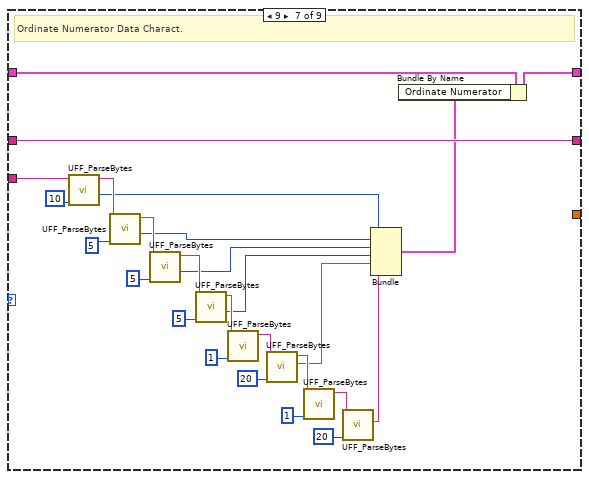
[diagram p12: hidden frame]
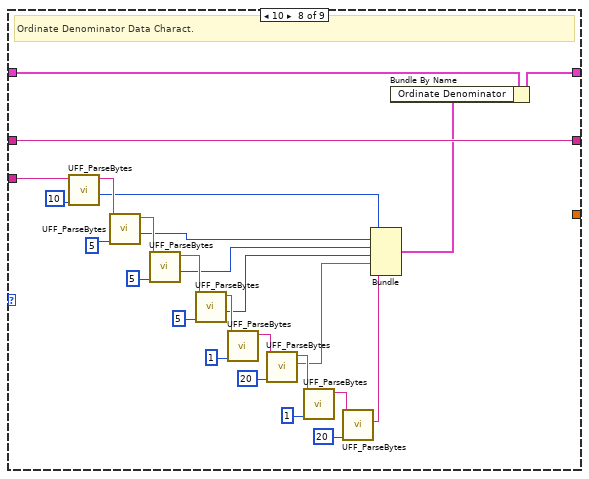
[diagram p13: hidden frame]
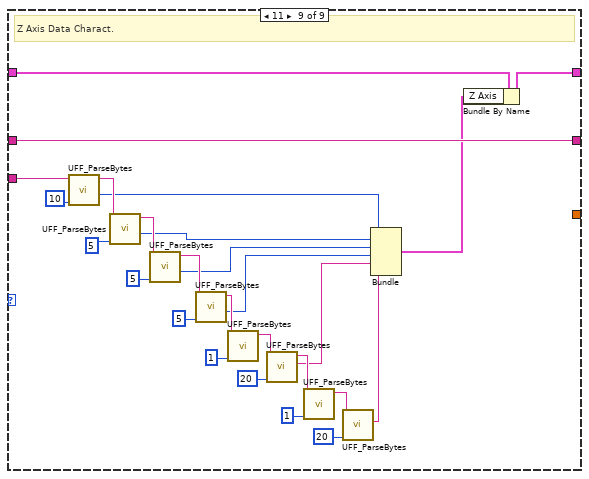
[diagram p14: hidden frame]
diagram:
  w8 = 1.25
  # "Name:   Function at Nodal DOF\nStatus: Current\nOwner:  Test\nRevision Date: 30-Jun-1999\n\n \n-----------------------------------------------------------------------\n \n         Record 1:     Format(80A1)\n                       Field 1    - ID Line 1\n \n                                                 NOTE\n \n                           ID Line 1 is generally  used  for  the  function\n                           description.\n \n \n         Record 2:     Format(80A1)\n                       Field 1    - ID Line 2\n \n         Record 3:     Format(80A1)\n                       Field 1    - ID Line 3\n \n                                                 NOTE\n \n                           ID Line 3 is generally used to identify when the\n                           function  was  created.  The date is in the form\n                           DD-MMM-YY, and the time is in the form HH:MM:SS,\n                           with a general Format(9A1,1X,8A1).\n \n \n         Record 4:     Format(80A1)\n                       Field 1    - ID Line 4\n \n         Record 5:     Format(80A1)\n                       Field 1    - ID Line 5\n \n         Record 6:     Format(2(I5,I10),2(1X,10A1,I10,I4))\n                                  DOF Identification\n                       Field 1    - Function Type\n                                    0 - General or Unknown\n                                    1 - Time Response\n                                    2 - Auto Spectrum\n                                    3 - Cross Spectrum\n                                    4 - Frequency Response Function\n                                    5 - Transmissibility\n                                    6 - Coherence\n                                    7 - Auto Correlation\n                                    8 - Cross Correlation\n                                    9 - Power Spectral Density (PSD)\n                                    10 - Energy Spectral Density (ESD)\n                                    11 - Probability Density Function\n                                    12 - Spectrum\n                                    13 - Cumulative Frequency Distribution\n                                    14 - Peaks Valley\n                                    15 - Stress/Cycles\n                                    16 - Strain/Cycles\n                                    17 - Orbit\n                                    18 - Mode Indicator Function\n                                    19 - Force Pattern\n                                    20 - Partial Power\n                                    21 - Partial Coherence\n                                    22 - Eigenvalue\n                                    23 - Eigenvector\n                                    24 - Shock Response Spectrum\n                                    25 - Finite Impulse Response Filter\n                                    26 - Multiple Coherence\n                                    27 - Order Function\n                                    28 - Phase Compensation\n                       Field 2    - Function Identification Number\n                       Field 3    - Version Number, or sequence number\n                       Field 4    - Load Case Identification Number\n                                    0 - Single Point Excitation\n                       Field 5    - Response Entity Name (\"NONE\" if unused)\n                       Field 6    - Response Node\n                       Field 7    - Response Direction\n                                     0 - Scalar\n                                     1 - +X Translation       4 - +X Rotation\n                                    -1 - -X Translation      -4 - -X Rotation\n                                     2 - +Y Translation       5 - +Y Rotation\n                                    -2 - -Y Translation      -5 - -Y Rotation\n                                     3 - +Z Translation       6 - +Z Rotation\n                                    -3 - -Z Translation      -6 - -Z Rotation\n                       Field 8    - Reference Entity Name (\"NONE\" if unused)\n                       Field 9    - Reference Node\n                       Field 10   - Reference Direction  (same as field 7)\n \n                                                 NOTE\n \n                           Fields 8, 9, and 10 are only relevant if field 4\n                           is zero.\n \n \n \n \n        Record 7:     Format(3I10,3E13.5)\n                                  Data Form\n                       Field 1    - Ordinate Data Type\n                                    2 - real, single precision\n                                    4 - real, double precision\n                                    5 - complex, single precision\n                                    6 - complex, double precision\n                       Field 2    - Number of data pairs for uneven  abscissa\n                                    spacing, or number of data values for even\n                                    abscissa spacing\n                       Field 3    - Abscissa Spacing\n                                    0 - uneven\n                                    1 - even (no abscissa values stored)\n                       Field 4    - Abscissa minimum (0.0 if spacing uneven)\n                       Field 5    - Abscissa increment (0.0 if spacing uneven)\n                       Field 6    - Z-axis value (0.0 if unused)\n \n         Record 8:     Format(I10,3I5,2(1X,20A1))\n                                  Abscissa Data Characteristics\n                       Field 1    - Specific Data Type\n                                    0 - unknown\n                                    1 - general\n                                    2 - stress\n                                    3 - strain\n                                    5 - temperature\n                                    6 - heat flux\n                                    8 - displacement\n                                    9 - reaction force\n                                    11 - velocity\n                                    12 - acceleration\n                                    13 - excitation force\n                                    15 - pressure\n                                    16 - mass\n                                    17 - time\n                                    18 - frequency\n                                    19 - rpm\n                                    20 - order\n                                    21 - sound pressure\n                                    22 - sound intensity\n                                    23 - sound power\n                       Field 2    - Length units exponent\n                       Field 3    - Force units exponent\n                       Field 4    - Temperature units exponent\n \n                                                 NOTE\n \n                           Fields 2, 3 and  4  are  relevant  only  if  the\n                           Specific Data Type is General, or in the case of\n                           ordinates, the response/reference direction is a\n                           scalar, or the functions are being used for\n                           nonlinear connectors in System Dynamics Analysis.\n                           See Addendum 'A' for the units exponent table.\n \n                       Field 5    - Axis label (\"NONE\" if not used)\n                       Field 6    - Axis units label (\"NONE\" if not used)\n \n                                                 NOTE\n \n                           If fields  5  and  6  are  supplied,  they  take\n                           precendence  over  program  generated labels and\n                           units.\n \n         Record 9:     Format(I10,3I5,2(1X,20A1))\n                       Ordinate (or ordinate numerator) Data Characteristics\n \n         Record 10:    Format(I10,3I5,2(1X,20A1))\n                       Ordinate Denominator Data Characteristics\n \n         Record 11:    Format(I10,3I5,2(1X,20A1))\n                       Z-axis Data Characteristics\n \n                                                 NOTE\n \n                           Records 9, 10, and 11 are  always  included  and\n                           have fields the same as record 8.  If records 10\n                           and 11 are not used, set field 1 to zero.\n \n\n \n         Record 12:\n                                   Data Values\n \n                         Ordinate            Abscissa\n             Case     Type     Precision     Spacing       Format\n           -------------------------------------------------------------\n               1      real      single        even         6E13.5\n               2      real      single       uneven        6E13.5\n               3     complex    single        even         6E13.5\n               4     complex    single       uneven        6E13.5\n               5      real      double        even         4E20.12\n               6      real      double       uneven     2(E13.5,E20.12)\n               7     complex    double        even         4E20.12\n               8     complex    double       uneven      E13.5,2E20.12\n           --------------------------------------------------------------\n \n                                          NOTE\n \n           See  Addendum  'B'  for  typical  FORTRAN   READ/WRITE\n           statements for each case.\n \n \n         General Notes:\n \n              1.  ID lines may not be blank.  If no  information  is  required,\n                  the word \"NONE\" must appear in columns 1 through 4.\n \n              2.  ID line 1 appears on plots in Finite Element Modeling and is\n                  used as the function description in System Dynamics Analysis.\n \n              3.  Dataloaders use the following ID line conventions\n                     ID Line 1 - Model Identification\n                     ID Line 2 - Run Identification\n                     ID Line 3 - Run Date and Time\n                     ID Line 4 - Load Case Name\n \n              4.  Coordinates codes from MODAL-PLUS and MODALX are decoded into\n                  node and direction.\n \n              5.  Entity names used in System Dynamics Analysis prior to I-DEAS\n                  Level 5 have a 4 character maximum. Beginning with Level 5,\n                  entity names will be ignored if this dataset is preceded by\n                  dataset 259. If no dataset 259 precedes this dataset, then the\n                  entity name will be assumed to exist in model bin number 1.\n \n              6.  Record 10 is ignored by System Dynamics Analysis unless load\n                  case = 0. Record 11 is always ignored by System Dynamics\n                  Analysis.\n \n              7.  In record 6, if the response or reference names are \"NONE\"\n                  and are not overridden by a dataset 259, but the correspond-\n                  ing node is non-zero, System Dynamics Analysis adds the node\n                  and direction to the function description if space is sufficie\n \n              8.  ID line 1 appears on XY plots in Test Data Analysis along\n                  with ID line 5 if it is defined.  If defined, the axis units\n                  labels also appear on the XY plot instead of the normal\n                  labeling based on the data type of the function.\n \n              9.  For functions used with nonlinear connectors in System\n                  Dynamics Analysis, the following requirements must be\n                  adhered to:\n \n                  a) Record 6: For a displacement-dependent function, the\n                     function type must be 0; for a frequency-dependent\n                     function, it must be 4. In either case, the load case\n                     identification number must be 0.\n \n                  b) Record 8: For a displacement-dependent function, the\n                     specific data type must be 8 and the length units\n                     exponent must be 0 or 1; for a frequency-dependent\n                     function, the specific data type must be 18 and the\n                     length units exponent must be 0. In either case, the\n                     other units exponents must be 0.\n \n                  c) Record 9: The specific data type must be 13. The\n                     temperature units exponent must be 0. For an ordinate\n                     numerator of force, the length and force units\n                     exponents must be 0 and 1, respectively. For an\n                     ordinate numerator of moment, the length and force\n                     units exponents must be 1 and 1, respectively.\n \n                  d) Record 10: The specific data type must be 8 for\n                     stiffness and hysteretic damping; it must be 11\n                     for viscous damping. For an ordinate denominator of\n                     translational displacement, the length units exponent\n                     must be 1; for a rotational displacement, it must\n                     be 0. The other units exponents must be 0.\n \n                  e) Dataset 217 must precede each function in order to\n                     define the function's usage (i.e. stiffness, viscous\n                     damping, hysteretic damping).\n \n \n\n                                       Addendum A\n \n         In order to correctly perform units  conversion,  length,  force,  and\n         temperature  exponents  must  be  supplied for a specific data type of\n         General; that is, Record 8 Field 1 = 1.  For example, if the  function\n         has  the  physical dimensionality of Energy (Force * Length), then the\n         required exponents would be as follows:\n \n                 Length = 1\n                 Force = 1          Energy = L * F\n                 Temperature = 0\n \n         Units exponents for the remaining specific data types  should  not  be\n         supplied.  The following exponents will automatically be used.\n \n \n                              Table - Unit Exponents\n              -------------------------------------------------------\n               Specific                   Direction\n                        ---------------------------------------------\n                 Data       Translational            Rotational\n                        ---------------------------------------------\n                 Type    Length  Force  Temp    Length  Force  Temp\n              -------------------------------------------------------\n                  0        0       0      0       0       0      0\n                  1             (requires input to fields 2,3,4)\n                  2       -2       1      0      -1       1      0\n                  3        0       0      0       0       0      0\n                  5        0       0      1       0       0      1\n                  6        1       1      0       1       1      0\n                  8        1       0      0       0       0      0\n                  9        0       1      0       1       1      0\n                 11        1       0      0       0       0      0\n                 12        1       0      0       0       0      0\n                 13        0       1      0       1       1      0\n                 15       -2       1      0      -1       1      0\n                 16       -1       1      0       1       1      0\n                 17        0       0      0       0       0      0\n                 18        0       0      0       0       0      0\n                 19        0       0      0       0       0      0\n              --------------------------------------------------------\n \n                                          NOTE\n \n                 Units exponents for scalar points are defined within\n                 System Analysis prior to reading this dataset.\n \n\n \n                                       Addendum B\n \n         There are 8 distinct  combinations  of  parameters  which  affect  the\n         details   of  READ/WRITE  operations.   The  parameters  involved  are\n         Ordinate Data Type, Ordinate Data  Precision,  and  Abscissa  Spacing.\n         Each  combination  is documented in the examples below.  In all cases,\n         the number of data values (for even abscissa spacing)  or  data  pairs\n         (for  uneven  abscissa  spacing)  is NVAL.  The abcissa is always real\n         single precision.  Complex double precision is  handled  by  two  real\n         double  precision  variables  (real  part  followed by imaginary part)\n         because most systems do not directly support complex double precision.\n \n         CASE 1\n \n         REAL\n         SINGLE PRECISION\n         EVEN SPACING\n \n           Order of data in file           Y1   Y2   Y3   Y4   Y5   Y6\n                                           Y7   Y8   Y9   Y10  Y11  Y12\n                                                      .\n                                                      .\n                                                      .\n           Input\n \n                     REAL Y(6)\n                       .\n                       .\n                       .\n                     NPRO=0\n                  10 READ(LUN,1000,ERR=  ,END=  )(Y(I),I=1,6)\n                1000 FORMAT(6E13.5)\n                     NPRO=NPRO+6\n                       .\n                       .    code to process these six values\n                       .\n                     IF(NPRO.LT.NVAL)GO TO 10\n                       .\n                       .   continued processing\n                       .\n \n           Output\n \n                     REAL Y(6)\n                       .\n                       .\n                       .\n                     NPRO=0\n                  10 CONTINUE\n                       .\n                       .    code to set up these six values\n                       .\n                     WRITE(LUN,1000,ERR=  )(Y(I),I=1,6)\n                1000 FORMAT(6E13.5)\n                     NPRO=NPRO+6\n \n                     IF(NPRO.LT.NVAL)GO TO 10\n                       .\n                       .   continued processing\n                       .\n \n         CASE 2\n \n         REAL\n         SINGLE PRECISION\n         UNEVEN SPACING\n \n           Order of data in file          X1   Y1   X2   Y2   X3   Y3\n                                          X4   Y4   X5   Y5   X6   Y6\n                                           .\n                                           .\n                                           .\n\n \n \n           Input\n \n                     REAL X(3),Y(3)\n                       .\n                       .\n                       .\n                     NPRO=0\n                  10 READ(LUN,1000,ERR=  ,END=  )(X(I),Y(I),I=1,3)\n                1000 FORMAT(6E13.5)\n                     NPRO=NPRO+3\n                       .\n                       .    code to process these three values\n                       .\n                     IF(NPRO.LT.NVAL)GO TO 10\n                       .\n                       .   continued processing\n                       .\n \n \n           Output\n \n                     REAL X(3),Y(3)\n                       .\n                       .\n                       .\n                     NPRO=0\n                  10 CONTINUE\n                       .\n                       .    code to set up these three values\n                       .\n                     WRITE(LUN,1000,ERR=  )(X(I),Y(I),I=1,3)\n                1000 FORMAT(6E13.5)\n                     NPRO=NPRO+3\n                     IF(NPRO.LT.NVAL)GO TO 10\n                       .\n                       .   continued processing\n                       .\n \n         CASE 3\n \n         COMPLEX\n         SINGLE PRECISION\n         EVEN SPACING\n \n           Order of data in file          RY1  IY1  RY2  IY2  RY3  IY3\n                                          RY4  IY4  RY5  IY5  RY6  IY6\n                                           .\n                                           .\n                                           .\n \n           Input\n \n                     COMPLEX Y(3)\n                       .\n                       .\n                       .\n                     NPRO=0\n                  10 READ(LUN,1000,ERR=  ,END=  )(Y(I),I=1,3)\n                1000 FORMAT(6E13.5)\n                     NPRO=NPRO+3\n                       .\n                       .    code to process these six values\n                       .\n                     IF(NPRO.LT.NVAL)GO TO 10\n                       .\n                       .   continued processing\n                       .\n \n \n           Output\n \n                     COMPLEX Y(3)\n                       .\n                       .\n                       .\n                     NPRO=0\n                  10 CONTINUE\n                       .\n                       .    code to set up these three values\n                       .\n                     WRITE(LUN,1000,ERR=  )(Y(I),I=1,3)\n                1000 FORMAT(6E13.5)\n                     NPRO=NPRO+3\n                     IF(NPRO.LT.NVAL)GO TO 10\n                       .\n                       .   continued processing\n                       .\n \n \n \n        CASE 4\n \n         COMPLEX\n         SINGLE PRECISION\n         UNEVEN SPACING\n \n           Order of data in file          X1   RY1  IY1  X2  RY2  IY2\n                                          X3   RY3  IY3  X4  RY4  IY4\n \n                                           .\n                                           .\n                                           .\n \n           Input\n \n                     REAL X(2)\n                     COMPLEX Y(2)\n                       .\n                       .\n                       .\n                     NPRO=0\n                  10 READ(LUN,1000,ERR=  ,END=  )(X(I),Y(I),I=1,2)\n                1000 FORMAT(6E13.5)\n                     NPRO=NPRO+2\n                       .\n                       .    code to process these two values\n                       .\n                     IF(NPRO.LT.NVAL)GO TO 10\n                       .\n                       .   continued processing\n                       .\n \n          Output\n \n                     REAL X(2)\n                     COMPLEX Y(2)\n                       .\n                       .\n                       .\n                     NPRO=0\n                  10 CONTINUE\n                       .\n                       .    code to set up these two values\n                       .\n                     WRITE(LUN,1000,ERR=  )(X(I),Y(I),I=1,2)\n                1000 FORMAT(6E13.5)\n                     NPRO=NPRO+2\n                     IF(NPRO.LT.NVAL)GO TO 10\n                       .\n                       .   continued processing\n                       .\n \n         CASE 5\n \n         REAL\n         DOUBLE PRECISION\n         EVEN SPACING\n \n           Order of data in file          Y1     Y2     Y3     Y4\n                                          Y5     Y6     Y7     Y8\n                                           .\n                                           .\n                                           .\n           Input\n \n                     DOUBLE PRECISION Y(4)\n                       .\n                       .\n                       .\n                     NPRO=0\n                  10 READ(LUN,1000,ERR=  ,END=  )(Y(I),I=1,4)\n                1000 FORMAT(4E20.12)\n                     NPRO=NPRO+4\n                       .\n                       .    code to process these four values\n                       .\n                     IF(NPRO.LT.NVAL)GO TO 10\n                       .\n                       .   continued processing\n                       .\n \n \n           Output\n \n                     DOUBLE PRECISION Y(4)\n                       .\n                       .\n                       .\n                     NPRO=0\n                  10 CONTINUE\n                       .\n                       .    code to set up these four values\n                       .\n                     WRITE(LUN,1000,ERR=  )(Y(I),I=1,4)\n                1000 FORMAT(4E20.12)\n                     NPRO=NPRO+4\n                     IF(NPRO.LT.NVAL)GO TO 10\n                       .\n                       .   continued processing\n                       .\n \n         CASE 6\n \n         REAL\n         DOUBLE PRECISION\n         UNEVEN SPACING\n \n           Order of data in file          X1   Y1     X2   Y2\n                                          X3   Y3     X4   Y4\n                                           .\n                                           .\n                                           .\n           Input\n \n                     REAL X(2)\n                     DOUBLE PRECISION Y(2)\n                       .\n                       .\n                       .\n                     NPRO=0\n                  10 READ(LUN,1000,ERR=  ,END=  )(X(I),Y(I),I=1,2)\n                1000 FORMAT(2(E13.5,E20.12))\n                     NPRO=NPRO+2\n                       .\n                       .    code to process these two values\n                       .\n                     IF(NPRO.LT.NVAL)GO TO 10\n                       .\n                       .   continued processing\n                       .\n \n           Output\n \n                     REAL X(2)\n                     DOUBLE PRECISION Y(2)\n                       .\n                       .\n                       .\n                     NPRO=0\n                  10 CONTINUE\n                       .\n                       .    code to set up these two values\n                       .\n                     WRITE(LUN,1000,ERR=  )(X(I),Y(I),I=1,2)\n                1000 FORMAT(2(E13.5,E20.12))\n                     NPRO=NPRO+2\n                     IF(NPRO.LT.NVAL)GO TO 10\n                       .\n                       .   continued processing\n                       .\n \n\n \n         CASE 7\n \n         COMPLEX\n         DOUBLE PRECISION\n         EVEN SPACING\n \n           Order of data in file          RY1    IY1    RY2    IY2\n                                          RY3    IY3    RY4    IY4\n                                           .\n                                           .\n                                           .\n \n           Input\n \n                     DOUBLE PRECISION Y(2,2)\n                       .\n                       .\n                       .\n                     NPRO=0\n                  10 READ(LUN,1000,ERR=  ,END=  )((Y(I,J),I=1,2),J=1,2)\n                1000 FORMAT(4E20.12)\n                     NPRO=NPRO+2\n                       .\n                       .    code to process these two values\n                       .\n                     IF(NPRO.LT.NVAL)GO TO 10\n                       .\n                       .   continued processing\n                       .\n \n           Output\n \n                     DOUBLE PRECISION Y(2,2)\n                       .\n                       .\n                       .\n                     NPRO=0\n                  10 CONTINUE\n                       .\n                       .    code to set up these two values\n                       .\n                     WRITE(LUN,1000,ERR=  )((Y(I,J),I=1,2),J=1,2)\n                1000 FORMAT(4E20.12)\n                     NPRO=NPRO+2\n                     IF(NPRO.LT.NVAL)GO TO 10\n                       .\n                       .   continued processing\n                       .\n         CASE 8\n \n         COMPLEX\n         DOUBLE PRECISION\n         UNEVEN SPACING\n \n           Order of data in file          X1   RY1    IY1\n                                          X2   RY2    IY2\n                                           .\n                                           .\n                                           .\n           Input\n \n                     REAL X\n                     DOUBLE PRECISION Y(2)\n                       .\n                       .\n                       .\n                     NPRO=0\n                  10 READ(LUN,1000,ERR=  ,END=  )(X,Y(I),I=1,2)\n                1000 FORMAT(E13.5,2E20.12)\n                     NPRO=NPRO+1\n                       .\n                       .    code to process this value\n                       .\n                     IF(NPRO.LT.NVAL)GO TO 10\n                       .\n                       .   continued processing\n                       .\n \n           Output\n \n                     REAL X\n                     DOUBLE PRECISION Y(2)\n                       .\n                       .\n                       .\n                     NPRO=0\n                  10 CONTINUE\n                       .\n                       .    code to set up this value\n                       .\n                     WRITE(LUN,1000,ERR=  )(X,Y(I),I=1,2)\n                1000 FORMAT(E13.5,2E20.12)\n                     NPRO=NPRO+1\n                     IF(NPRO.LT.NVAL)GO TO 10\n                       .\n                       .   continued processing\n                       .\n \n-----------------------------------------------------------------------"
  n1 = local read "DataSet"() -> (w5:T1)
  n2 = for {
    tunnel: "array" -> [w18] mode=indexing
    shift-right: [w16] -> w10
    shift-left: "" -> [w17]
    tunnel: [w15] -> w6 mode=concatenating
    shift-right: [w13] -> w3
    shift-left: w5 -> [w14]
    i -> [w19]
    n3 = case shown="Default" w19 {
      tunnel: w18 -> [w20 w74 w77 w116 w138 w164 w190 w216 w242]
      tunnel: w17 -> [w23 w73 w79 w117 w139 w165 w191 w217 w243]
      tunnel: [w23 w73 w78 w117 w139 w165 w191 w217 w243] -> w16
      tunnel: [w22 _ _ _ _ _ _ _ _] -> w15
      tunnel: w14 -> [w21 w71 w75 w82 w118 w141 w167 w193 w219]
      tunnel: [w21 w71 w75 w81 w119 w140 w166 w194 w218] -> w13
      frame Default {
        # "Data"
        n4 = case shown="Default" w20 {
          tunnel: w20 -> [_ w30]
          tunnel: [cdb[] [] w25] -> w22
          tunnel: w21 -> [_ w29]
          frame "" {
          }
          frame Default {
            n5 = Unbundle By Name(w29) -> ("Data Form.Ordinate Data Type"=w32:T2, "Data Form.Abscissa Spacing"=w31:enum16{"Uneven", "Even"})
            n6 = case shown="\"Real SGL\", \"Complex SGL\"" w32 {
              tunnel: [dbl[] [] w36 w44] -> w28
              tunnel: w31 -> [_ _ w43]
              tunnel: w30 -> [_ w34 w42]
              frame Default {
              }
              frame "Real SGL", "Complex SGL" {
                n7 = for {
                  N: 6 -> [_]
                  tunnel: [w40] -> w36 mode=indexing if=w37
                  shift-right: [w39] -> _
                  shift-left: w34 -> [w41]
                  n8 = call "UFF_ParseBytes.vi"("length"=13, "String in"=w41) -> ("number"=w40:dbl, "String out"=w39:string, "no error"=w37:bool)  [unwired: 5 in, 2 out]
                }
              }
              frame "Real DBL", "Complex DBL" {
                n9 = case shown="\"Uneven\"" w43 {
                  tunnel: [w47 w55] -> w44
                  tunnel: w42 -> [w45 w53]
                  frame "Even" {
                    n10 = for {
                      N: 4 -> [_]
                      tunnel: [w51] -> w47 mode=indexing if=w48
                      shift-right: [w50] -> _
                      shift-left: w45 -> [w52]
                      n11 = call "UFF_ParseBytes.vi"("length"=20, "String in"=w52) -> ("number"=w51:dbl, "String out"=w50:string, "no error"=w48:bool)  [unwired: 5 in, 2 out]
                    }
                  }
                  frame "Uneven" {
                    n12 = for {
                      N: 4 -> [_]
                      tunnel: [w59] -> w55 mode=indexing if=w56
                      shift-right: [w58] -> _
                      shift-left: w53 -> [w60]
                      i -> [w57]
                      n13 = case shown="0, 2, Default" w57 {
                        tunnel: w60 -> [w65 w70]
                        tunnel: [w64 w69] -> w59
                        tunnel: [w63 w68] -> w58
                        tunnel: [w61 w66] -> w56
                        frame 1, 3 {
                          n14 = call "UFF_ParseBytes.vi"("length"=20, "String in"=w65) -> ("number"=w64:dbl, "String out"=w63:string, "no error"=w61:bool)  [unwired: 5 in, 2 out]
                        }
                        frame 0, 2, Default {
                          n15 = call "UFF_ParseBytes.vi"("length"=13, "String in"=w70) -> ("number"=w69:dbl, "String out"=w68:string, "no error"=w66:bool)  [unwired: 5 in, 2 out]
                        }
                      }
                    }
                  }
                }
              }
            }
            n16 = Decimate 1D Array(w28) -> (w26:dbl[], w27:dbl[])
            n17 = Re/Im To Complex(1:w27, 2:w26) -> (0:w25:cdb[])
          }
        }
      }
      frame 0 {
        # "Don't Know"
        n18 = Decimal String To Number(string=w74) -> (number=→"UF Dataset type":i32)  [unwired: 2 in, 1 out]
      }
      frame 1..5 {
        # "ID Lines (3 = time)"
        n19 = Concatenate Strings(w79, w77, "\n" ("string")) -> (w78:string)
      }
      frame 6 {
        # "DOF ID"
        n20 = call "UFF_ParseBytes.vi"("length"=5 ("length (rest)"), "String in"=w116) -> ("Value"=w92:i32, "String out"=w114:string)  [unwired: 5 in, 3 out]
        n21 = call "UFF_ParseBytes.vi"("length"=10 ("length (rest)"), "String in"=w114) -> ("Value"=w91:i32, "String out"=w111:string)  [unwired: 5 in, 3 out]
        n22 = call "UFF_ParseBytes.vi"("length"=5 ("length (rest)"), "String in"=w111) -> ("Value"=w90:i32, "String out"=w108:string)  [unwired: 5 in, 3 out]
        n23 = call "UFF_ParseBytes.vi"("length"=10 ("length (rest)"), "String in"=w108) -> ("Value"=w89:i32, "String out"=w107:string)  [unwired: 5 in, 3 out]
        n24 = call "UFF_ParseBytes.vi"("length"=1 ("length (rest)"), "String in"=w107) -> ("String out"=w105:string)  [unwired: 5 in, 4 out]
        n25 = call "UFF_ParseBytes.vi"("length"=10 ("length (rest)"), "String in"=w105) -> ("Subset"=w88:string, "String out"=w103:string)  [unwired: 5 in, 3 out]
        n26 = call "UFF_ParseBytes.vi"("length"=10 ("length (rest)"), "String in"=w103) -> ("Value"=w87:i32, "String out"=w101:string)  [unwired: 5 in, 3 out]
        n27 = call "UFF_ParseBytes.vi"("length"=4 ("length (rest)"), "String in"=w101) -> ("Value"=w86:i32, "String out"=w93:string)  [unwired: 5 in, 3 out]
        n28 = call "UFF_ParseBytes.vi"("length"=1 ("length (rest)"), "String in"=w93) -> ("String out"=w96:string)  [unwired: 5 in, 4 out]
        n29 = call "UFF_ParseBytes.vi"("length"=10 ("length (rest)"), "String in"=w96) -> ("Subset"=w85:string, "String out"=w98:string)  [unwired: 5 in, 3 out]
        n30 = call "UFF_ParseBytes.vi"("length"=10 ("length (rest)"), "String in"=w98) -> ("Value"=w84:i32, "String out"=w100:string)  [unwired: 5 in, 3 out]
        n31 = call "UFF_ParseBytes.vi"("length"=4 ("length (rest)"), "String in"=w100) -> ("Value"=w83:i32)  [unwired: 5 in, 4 out]
        n32 = Bundle("Value"=w92, "Value"=w91, "Value"=w90, "Value"=w89, "Subset"=w88, "Value"=w87, "Value"=w86, "Subset"=w85, "Value"=w84, "Value"=w83) -> (w80:T3)  [unwired: 1 in]
        n33 = Bundle By Name(cluster=w82, "DOF ID"=w80) -> (w81:T1)
      }
      frame 7 {
        # "Data Form"
        n34 = call "UFF_ParseBytes.vi"("length"=10 ("length (rest)"), "String in"=w138) -> ("Value"=w126:i32, "String out"=w136:string)  [unwired: 5 in, 3 out]
        n35 = call "UFF_ParseBytes.vi"("length"=10 ("length (rest)"), "String in"=w136) -> ("Value"=w125:i32, "String out"=w133:string)  [unwired: 5 in, 3 out]
        n36 = call "UFF_ParseBytes.vi"("length"=10 ("length (rest)"), "String in"=w133) -> ("Value"=w124:i32, "String out"=w131:string)  [unwired: 5 in, 3 out]
        n37 = call "UFF_ParseBytes.vi"("length"=13 ("length (rest)"), "String in"=w131) -> ("number"=w123:dbl, "String out"=w128:string)  [unwired: 5 in, 3 out]
        n38 = call "UFF_ParseBytes.vi"("length"=13 ("length (rest)"), "String in"=w128) -> ("number"=w122:dbl, "String out"=w127:string)  [unwired: 5 in, 3 out]
        n39 = call "UFF_ParseBytes.vi"("length"=13 ("length (rest)"), "String in"=w127) -> ("number"=w121:dbl)  [unwired: 5 in, 4 out]
        n40 = Bundle("Value"=w126, "Value"=w125, "Value"=w124, "number"=w123, "number"=w122, "number"=w121) -> (w120:T4)  [unwired: 1 in]
        n41 = Bundle By Name(cluster=w118, "Data Form"=w120) -> (w119:T1)
      }
      frame 8 {
        # "Abscissa Data Charact."
        n42 = call "UFF_ParseBytes.vi"("length"=10 ("length (rest)"), "String in"=w164) -> ("Value"=w148:i32, "String out"=w162:string)  [unwired: 5 in, 3 out]
        n43 = call "UFF_ParseBytes.vi"("length"=5 ("length (rest)"), "String in"=w162) -> ("Value"=w147:i32, "String out"=w159:string)  [unwired: 5 in, 3 out]
        n44 = call "UFF_ParseBytes.vi"("length"=5 ("length (rest)"), "String in"=w159) -> ("Value"=w146:i32, "String out"=w157:string)  [unwired: 5 in, 3 out]
        n45 = call "UFF_ParseBytes.vi"("length"=5 ("length (rest)"), "String in"=w157) -> ("Value"=w145:i32, "String out"=w154:string)  [unwired: 5 in, 3 out]
        n46 = call "UFF_ParseBytes.vi"("length"=1 ("length (rest)"), "String in"=w154) -> ("String out"=w153:string)  [unwired: 5 in, 4 out]
        n47 = call "UFF_ParseBytes.vi"("length"=20 ("length (rest)"), "String in"=w153) -> ("Subset"=w144:string, "String out"=w150:string)  [unwired: 5 in, 3 out]
        n48 = call "UFF_ParseBytes.vi"("length"=1 ("length (rest)"), "String in"=w150) -> ("String out"=w149:string)  [unwired: 5 in, 4 out]
        n49 = call "UFF_ParseBytes.vi"("length"=20 ("length (rest)"), "String in"=w149) -> ("Subset"=w143:string)  [unwired: 5 in, 4 out]
        n50 = Bundle("Value"=w148, "Value"=w147, "Value"=w146, "Value"=w145, "Subset"=w144, "Subset"=w143) -> (w142:T5)  [unwired: 1 in]
        n51 = Bundle By Name(cluster=w141, "Abscissa"=w142) -> (w140:T1)
      }
      frame 9 {
        # "Ordinate Numerator Data Charact."
        n52 = call "UFF_ParseBytes.vi"("length"=10 ("length (rest)"), "String in"=w190) -> ("Value"=w174:i32, "String out"=w188:string)  [unwired: 5 in, 3 out]
        n53 = call "UFF_ParseBytes.vi"("length"=5 ("length (rest)"), "String in"=w188) -> ("Value"=w173:i32, "String out"=w185:string)  [unwired: 5 in, 3 out]
        n54 = call "UFF_ParseBytes.vi"("length"=5 ("length (rest)"), "String in"=w185) -> ("Value"=w172:i32, "String out"=w183:string)  [unwired: 5 in, 3 out]
        n55 = call "UFF_ParseBytes.vi"("length"=5 ("length (rest)"), "String in"=w183) -> ("Value"=w171:i32, "String out"=w180:string)  [unwired: 5 in, 3 out]
        n56 = call "UFF_ParseBytes.vi"("length"=1 ("length (rest)"), "String in"=w180) -> ("String out"=w179:string)  [unwired: 5 in, 4 out]
        n57 = call "UFF_ParseBytes.vi"("length"=20 ("length (rest)"), "String in"=w179) -> ("Subset"=w170:string, "String out"=w176:string)  [unwired: 5 in, 3 out]
        n58 = call "UFF_ParseBytes.vi"("length"=1 ("length (rest)"), "String in"=w176) -> ("String out"=w175:string)  [unwired: 5 in, 4 out]
        n59 = call "UFF_ParseBytes.vi"("length"=20 ("length (rest)"), "String in"=w175) -> ("Subset"=w169:string)  [unwired: 5 in, 4 out]
        n60 = Bundle("Value"=w174, "Value"=w173, "Value"=w172, "Value"=w171, "Subset"=w170, "Subset"=w169) -> (w168:T5)  [unwired: 1 in]
        n61 = Bundle By Name(cluster=w167, "Ordinate Numerator"=w168) -> (w166:T1)
      }
      frame 10 {
        # "Ordinate Denominator Data Charact."
        n62 = call "UFF_ParseBytes.vi"("length"=10 ("length (rest)"), "String in"=w216) -> ("Value"=w200:i32, "String out"=w214:string)  [unwired: 5 in, 3 out]
        n63 = call "UFF_ParseBytes.vi"("length"=5 ("length (rest)"), "String in"=w214) -> ("Value"=w199:i32, "String out"=w211:string)  [unwired: 5 in, 3 out]
        n64 = call "UFF_ParseBytes.vi"("length"=5 ("length (rest)"), "String in"=w211) -> ("Value"=w198:i32, "String out"=w209:string)  [unwired: 5 in, 3 out]
        n65 = call "UFF_ParseBytes.vi"("length"=5 ("length (rest)"), "String in"=w209) -> ("Value"=w197:i32, "String out"=w206:string)  [unwired: 5 in, 3 out]
        n66 = call "UFF_ParseBytes.vi"("length"=1 ("length (rest)"), "String in"=w206) -> ("String out"=w205:string)  [unwired: 5 in, 4 out]
        n67 = call "UFF_ParseBytes.vi"("length"=20 ("length (rest)"), "String in"=w205) -> ("Subset"=w196:string, "String out"=w202:string)  [unwired: 5 in, 3 out]
        n68 = call "UFF_ParseBytes.vi"("length"=1 ("length (rest)"), "String in"=w202) -> ("String out"=w201:string)  [unwired: 5 in, 4 out]
        n69 = call "UFF_ParseBytes.vi"("length"=20 ("length (rest)"), "String in"=w201) -> ("Subset"=w195:string)  [unwired: 5 in, 4 out]
        n70 = Bundle("Value"=w200, "Value"=w199, "Value"=w198, "Value"=w197, "Subset"=w196, "Subset"=w195) -> (w192:T5)  [unwired: 1 in]
        n71 = Bundle By Name(cluster=w193, "Ordinate Denominator"=w192) -> (w194:T1)
      }
      frame 11 {
        # "Z Axis Data Charact."
        n72 = call "UFF_ParseBytes.vi"("length"=10 ("length (rest)"), "String in"=w242) -> ("Value"=w226:i32, "String out"=w240:string)  [unwired: 5 in, 3 out]
        n73 = call "UFF_ParseBytes.vi"("length"=5 ("length (rest)"), "String in"=w240) -> ("Value"=w225:i32, "String out"=w237:string)  [unwired: 5 in, 3 out]
        n74 = call "UFF_ParseBytes.vi"("length"=5 ("length (rest)"), "String in"=w237) -> ("Value"=w224:i32, "String out"=w235:string)  [unwired: 5 in, 3 out]
        n75 = call "UFF_ParseBytes.vi"("length"=5 ("length (rest)"), "String in"=w235) -> ("Value"=w223:i32, "String out"=w232:string)  [unwired: 5 in, 3 out]
        n76 = call "UFF_ParseBytes.vi"("length"=1 ("length (rest)"), "String in"=w232) -> ("String out"=w231:string)  [unwired: 5 in, 4 out]
        n77 = call "UFF_ParseBytes.vi"("length"=20 ("length (rest)"), "String in"=w231) -> ("Subset"=w222:string, "String out"=w228:string)  [unwired: 5 in, 3 out]
        n78 = call "UFF_ParseBytes.vi"("length"=1 ("length (rest)"), "String in"=w228) -> ("String out"=w227:string)  [unwired: 5 in, 4 out]
        n79 = call "UFF_ParseBytes.vi"("length"=20 ("length (rest)"), "String in"=w227) -> ("Subset"=w221:string)  [unwired: 5 in, 4 out]
        n80 = Bundle("Value"=w226, "Value"=w225, "Value"=w224, "Value"=w223, "Subset"=w222, "Subset"=w221) -> (w220:T5)  [unwired: 1 in]
        n81 = Bundle By Name(cluster=w219, "Z Axis"=w220) -> (w218:T1)
      }
    }
  }
  n82 = call <vilib>:"Trim Whitespace.vi"("string"=w10) -> ("trimmed string"=w4:string)  [unwired: 1 in]
  n83 = Array Size(array=w6) -> (size(s)=→"size(s)":i32)
  n84 = Complex To Polar(r * e^(i*theta)=w6) -> (r=w7:dbl[])  [unwired: 1 out]
  n85 = Bundle(w8, w8, w7) -> (w1:cluster{dbl, dbl, dbl[]})  [unwired: 1 in]
  n86 = Bundle By Name(cluster=w3, "Header"=w4, "Data"=w1) -> (→"DataSet":T1)
